vi "Bode plot.vi"(11 "input Bode plot":string) -> (0 "error out":errorcluster, 3 "Bode plot":dbl[][](graph))   [LabVIEW 2020, in "FBN_LATM.lvlib"]
uses:
  FBN_LATM.lvlib
  c2d5c92c-7b70-4316-925e-13b53ebf1ded.vi
  <vilib>/Array/Sort 2D Array - Pop Stack.vi
  <vilib>/Array/Sort 2D Array - Push Stack.vi
  c2d5c92c-7b70-4316-925e-13b53ebf1ded.vi/269d4b3b-47f5-49e3-8884-44851e4dd9d5.vi
  c2d5c92c-7b70-4316-925e-13b53ebf1ded.vi/6d99389c-673d-4efb-bf33-19b32bcf4cf8.vi
  <vilib>/regexp/Match Regular Expression.xnode
panel:
  out "XY Graph":T1(graph)
  out "PosAmpVsCur":dbl[](array[numeric])
  out "PosAmpVsPWM":dbl[](array[numeric])
  out "FreqHz":dbl[](array[numeric])
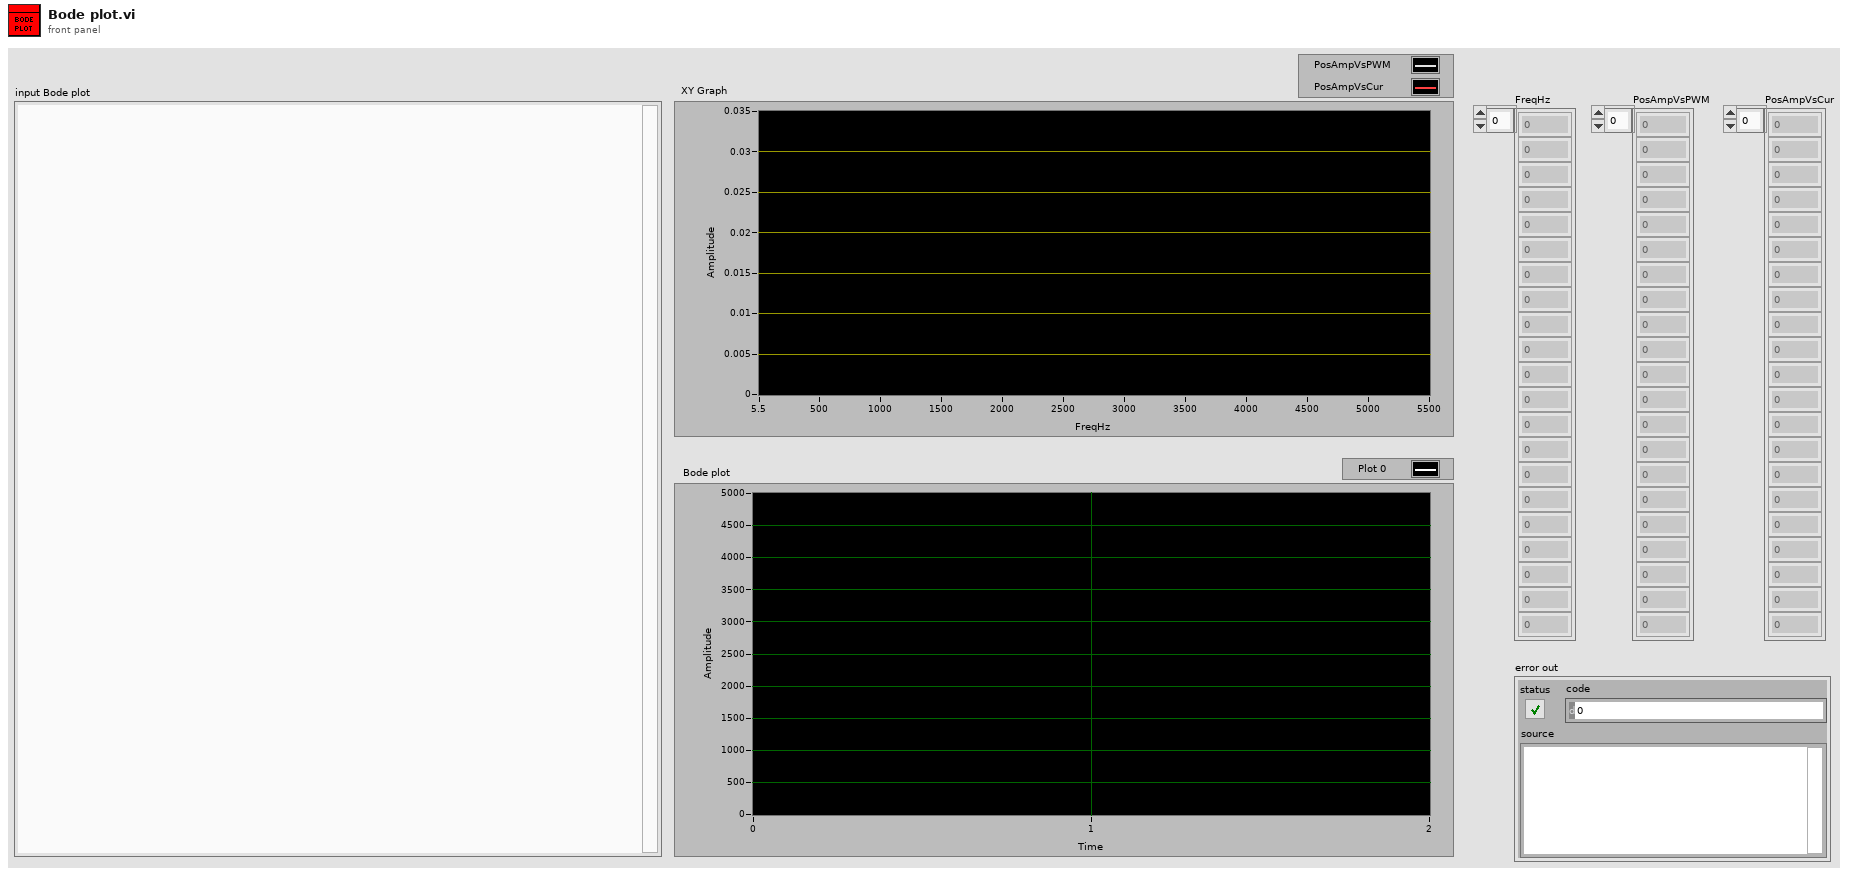
[diagram p1: front panel]
types:
  T1 = cluster{"sorted 2D array":dbl[], "sorted 2D array":dbl[]}[]
  T2 = cluster{"sorted 2D array":dbl[], "sorted 2D array":dbl[]}
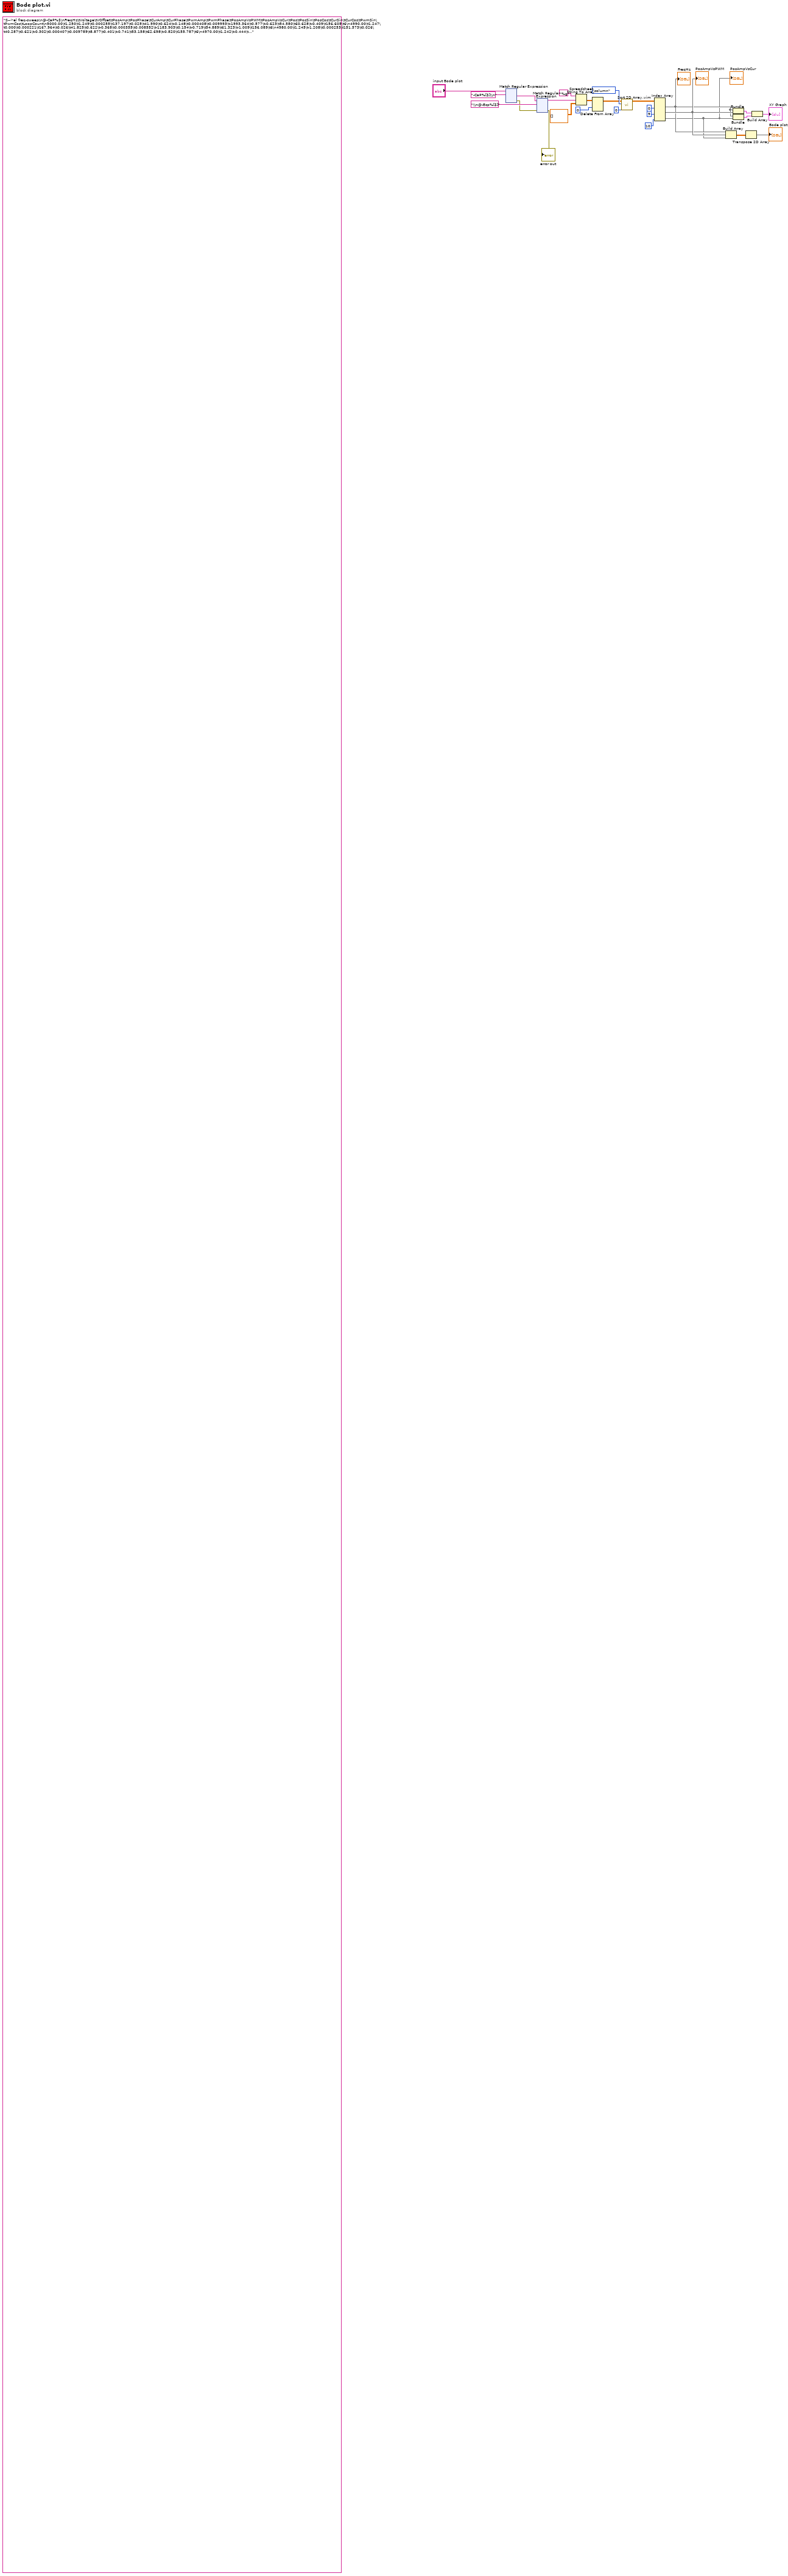
[diagram p0: block diagram]
diagram:
  (unwired) "S-->el freq-sweep\n@-CaP%$\nFreqHz\tVoltage\tVOffset\tPosAmp\tPosPhase\tCurAmp\tCurPhase\tPwmAmp\tPwmPhase\tPosAmpVsPWM\tPosAmpVsCur\tPos\tPosSin\tPosCos\tCurSin\tCurCos\tPwmSin\tPwmCos\tLoopCount\n5000.00\t1.250\t1.249\t0.000255\t137.197\t0.025\t41.990\t0.624\t-0.148\t0.000408\t0.009993\t-1993.364\t0.577\t-0.623\t54.580\t60.628\t-0.409\t156.605\t6\n4990.00\t1.247\t0.000\t0.000221\t167.964\t0.026\t41.825\t0.622\t-0.368\t0.000355\t0.008552\t-1183.903\t0.154\t-0.719\t54.889\t61.323\t-1.009\t156.089\t6\n4980.00\t1.245\t-1.208\t0.000253\t151.573\t0.026\t40.287\t0.621\t-0.302\t0.000407\t0.009789\t8.877\t0.401\t-0.741\t53.158\t62.698\t-0.820\t155.787\t6\n4970.00\t1.242\t-0.444\t0.000163\t148.359\t0.025\t42.056\t0.622\t-0.280\t0.000262\t0.006393\t355.367\t0.285\t-0.462\t54.627\t60.538\t-0.755\t155.800\t6\n4960.00\t1.240\t0.593\t0.000166\t155.248\t0.025\t42.473\t0.620\t-0.313\t0.000268\t0.006519\t341.746\t0.232\t-0.503\t55.286\t60.379\t-0.849\t155.524\t6\n4950.00\t1.237\t-0.866\t0.000154\t154.869\t0.026\t41.006\t0.618\t-0.264\t0.000248\t0.005952\t209.748\t0.218\t-0.464\t54.012\t62.121\t-0.713\t155.158\t6\n4940.00\t1.235\t-0.704\t0.000128\t155.479\t0.025\t41.111\t0.617\t-0.428\t0.000208\t0.005032\t31.794\t0.177\t-0.389\t53.478\t61.286\t-1.155\t154.830\t6\n4930.00\t1.232\t-1.089\t0.000129\t161.532\t0.025\t40.919\t0.615\t-0.330\t0.000209\t0.005050\t8.451\t0.136\t-0.407\t53.623\t61.863\t-0.891\t154.383\t6\n4920.00\t1.230\t-0.495\t0.000107\t155.632\t0.025\t41.869\t0.615\t-0.423\t0.000174\t0.004245\t-76.715\t0.147\t-0.325\t54.031\t60.266\t-1.137\t154.363\t6\n4910.00\t1.227\t1.228\t0.000117\t179.780\t0.026\t42.759\t0.613\t-0.297\t0.000191\t0.004534\t-61.266\t0.002\t-0.390\t55.773\t60.312\t-0.798\t153.814\t6\n4900.00\t1.225\t1.222\t0.000110\t169.025\t0.025\t41.786\t0.612\t-0.346\t0.000179\t0.004351\t-4.380\t0.070\t-0.358\t53.772\t60.160\t-0.925\t153.416\t6\n4890.00\t1.222\t0.000\t0.000144\t178.325\t0.026\t41.468\t0.610\t-0.324\t0.000236\t0.005571\t15.940\t0.014\t-0.479\t54.450\t61.610\t-0.860\t152.959\t6\n4880.00\t1.220\t1.126\t0.000127\t-174.326\t0.025\t41.984\t0.609\t-0.297\t0.000209\t0.004997\t20.182\t-0.042\t-0.422\t54.531\t60.584\t-0.787\t152.760\t6\n4870.00\t1.217\t1.038\t0.000151\t-172.441\t0.026\t42.028\t0.608\t-0.231\t0.000247\t0.005764\t16.908\t-0.066\t-0.498\t55.731\t61.821\t-0.608\t152.596\t6\n4860.00\t1.215\t0.900\t0.000139\t-176.287\t0.025\t41.808\t0.607\t-0.313\t0.000229\t0.005454\t41.706\t-0.030\t-0.462\t54.530\t60.955\t-0.826\t152.379\t6\n4850.00\t1.212\t-0.699\t0.000138\t-165.927\t0.025\t42.484\t0.605\t-0.258\t0.000229\t0.005423\t-5.301\t-0.112\t-0.447\t55.232\t60.289\t-0.682\t151.793\t6\n4840.00\t1.210\t-0.626\t0.000141\t-170.744\t0.026\t42.440\t0.605\t-0.324\t0.000232\t0.005388\t1.882\t-0.075\t-0.463\t56.283\t61.539\t-0.861\t151.883\t6\n4830.00\t1.207\t1.147\t0.000127\t-154.589\t0.025\t42.709\t0.603\t-0.385\t0.000211\t0.004990\t-23.980\t-0.182\t-0.383\t55.051\t59.628\t-1.015\t151.262\t6\n4820.00\t1.205\t0.049\t0.000151\t-162.762\t0.026\t43.033\t0.603\t-0.275\t0.000251\t0.005867\t31.689\t-0.150\t-0.482\t56.139\t60.142\t-0.720\t151.194\t6\n4810.00\t1.202\t-1.186\t0.000142\t-162.048\t0.025\t42.352\t0.601\t-0.412\t0.000236\t0.005624\t21.486\t-0.145\t-0.449\t54.368\t59.627\t-1.089\t150.646\t6\n4800.00\t1.200\t0.196\t0.000150\t-160.373\t0.025\t42.671\t0.600\t-0.269\t0.000249\t0.005866\t33.700\t-0.168\t-0.469\t55.084\t59.751\t-0.698\t150.332\t6\n4790.00\t1.197\t1.095\t0.000173\t-160.378\t0.026\t42.188\t0.597\t-0.269\t0.000290\t0.006714\t10.971\t-0.194\t-0.544\t55.137\t60.813\t-0.701\t149.884\t6\n4780.00\t1.195\t0.835\t0.000152\t-166.388\t0.025\t42.572\t0.597\t-0.291\t0.000254\t0.006026\t-16.344\t-0.119\t-0.491\t54.566\t59.388\t-0.767\t149.810\t6\n4770.00\t1.192\t-0.744\t0.000145\t-156.808\t0.025\t42.880\t0.597\t-0.346\t0.000242\t0.005678\t-13.537\t-0.190\t-0.444\t55.737\t60.020\t-0.905\t149.599\t6\n4760.00\t1.190\t-0.695\t0.000167\t-158.434\t0.026\t42.962\t0.595\t-0.286\t0.000281\t0.006482\t8.466\t-0.205\t-0.518\t56.481\t60.655\t-0.745\t149.185\t6\n4750.00\t1.187\t-1.041\t0.000176\t-159.659\t0.026\t43.500\t0.593\t-0.214\t0.000296\t0.006724\t-22.996\t-0.204\t-0.549\t57.545\t60.632\t-0.555\t148.691\t6\n4740.00\t1.185\t1.182\t0.000181\t-163.098\t0.026\t42.984\t0.592\t-0.231\t0.000306\t0.007017\t0.871\t-0.175\t-0.577\t56.165\t60.271\t-0.599\t148.323\t6\n4730.00\t1.183\t-1.161\t0.000143\t-157.346\t0.025\t44.495\t0.592\t-0.214\t0.000241\t0.005605\t30.673\t-0.183\t-0.440\t56.806\t57.809\t-0.556\t148.407\t6\n4720.00\t1.180\t0.115\t0.000160\t-163.207\t0.025\t43.731\t0.590\t-0.258\t0.000272\t0.006294\t2.617\t-0.155\t-0.512\t56.135\t58.670\t-0.671\t148.080\t6\n4710.00\t1.178\t0.000\t0.000164\t-164.745\t0.025\t44.121\t0.590\t-0.143\t0.000277\t0.006497\t-8.059\t-0.143\t-0.526\t56.342\t58.084\t-0.362\t147.814\t6\n4700.00\t1.175\t-1.164\t0.000155\t-156.242\t0.025\t43.720\t0.587\t-0.346\t0.000263\t0.006062\t3.469\t-0.208\t-0.471\t56.345\t58.904\t-0.886\t147.353\t6\n4690.00\t1.173\t0.000\t0.000177\t-164.910\t0.025\t42.056\t0.587\t-0.214\t0.000302\t0.006960\t-3.623\t-0.154\t-0.571\t54.614\t60.519\t-0.544\t147.385\t6\n4680.00\t1.170\t0.853\t0.000131\t-159.088\t0.025\t43.242\t0.585\t-0.417\t0.000223\t0.005127\t-1.643\t-0.156\t-0.407\t55.531\t59.054\t-1.064\t146.772\t6\n4670.00\t1.168\t-0.688\t0.000177\t-155.803\t0.025\t43.325\t0.583\t-0.236\t0.000304\t0.006948\t-3.205\t-0.242\t-0.538\t55.830\t59.196\t-0.599\t146.292\t6\n4660.00\t1.165\t-1.018\t0.000160\t-154.545\t0.025\t42.720\t0.583\t-0.313\t0.000275\t0.006374\t24.831\t-0.230\t-0.483\t54.934\t59.478\t-0.800\t146.112\t6\n4650.00\t1.163\t0.178\t0.000158\t-149.579\t0.026\t42.951\t0.581\t-0.417\t0.000272\t0.006128\t7.446\t-0.267\t-0.454\t56.012\t60.168\t-1.062\t145.766\t6\n4640.00\t1.160\t0.094\t0.000141\t-155.621\t0.025\t44.028\t0.580\t-0.406\t0.000243\t0.005599\t5.202\t-0.194\t-0.428\t55.760\t57.666\t-1.032\t145.551\t6\n4630.00\t1.158\t0.103\t0.000150\t-156.423\t0.025\t43.209\t0.579\t-0.341\t0.000259\t0.005887\t16.681\t-0.200\t-0.458\t55.817\t59.432\t-0.868\t145.294\t6\n4620.00\t1.155\t1.155\t0.000182\t-153.858\t0.026\t42.715\t0.578\t-0.297\t0.000315\t0.007058\t46.128\t-0.268\t-0.545\t55.730\t60.355\t-0.745\t144.788\t6\n4610.00\t1.153\t-0.619\t0.000159\t-155.132\t0.025\t44.764\t0.577\t-0.302\t0.000276\t0.006331\t16.596\t-0.224\t-0.482\t56.336\t56.801\t-0.757\t144.661\t6\n4600.00\t1.150\t-0.613\t0.000185\t-157.214\t0.025\t44.621\t0.575\t-0.319\t0.000323\t0.007276\t-14.436\t-0.239\t-0.570\t57.219\t57.971\t-0.808\t144.317\t6\n4590.00\t1.148\t0.831\t0.000185\t-148.211\t0.025\t45.093\t0.574\t-0.253\t0.000323\t0.007352\t22.962\t-0.325\t-0.524\t57.075\t56.877\t-0.636\t143.873\t6\n4580.00\t1.145\t0.899\t0.000161\t-151.941\t0.025\t44.247\t0.573\t-0.352\t0.000281\t0.006315\t26.916\t-0.253\t-0.474\t56.586\t58.077\t-0.883\t143.620\t6\n4570.00\t1.143\t0.000\t0.000167\t-156.423\t0.025\t44.094\t0.571\t-0.280\t0.000292\t0.006714\t12.777\t-0.222\t-0.510\t55.435\t57.206\t-0.698\t143.261\t6\n4560.00\t1.140\t1.140\t0.000178\t-148.870\t0.025\t45.143\t0.570\t-0.291\t0.000312\t0.007051\t-20.910\t-0.306\t-0.506\t57.204\t56.911\t-0.722\t143.006\t6\n4550.00\t1.138\t0.206\t0.000173\t-156.907\t0.025\t43.912\t0.569\t-0.368\t0.000304\t0.006781\t-28.046\t-0.226\t-0.530\t56.208\t58.365\t-0.921\t142.743\t6\n4540.00\t1.135\t-1.106\t0.000174\t-152.292\t0.025\t44.253\t0.568\t-0.357\t0.000306\t0.006992\t4.846\t-0.270\t-0.513\t55.734\t57.196\t-0.887\t142.371\t6\n4530.00\t1.133\t-0.389\t0.000175\t-148.788\t0.025\t45.192\t0.567\t-0.313\t0.000308\t0.006846\t23.396\t-0.302\t-0.498\t57.768\t57.377\t-0.769\t142.138\t6\n4520.00\t1.130\t-1.108\t0.000164\t-151.523\t0.025\t45.088\t0.565\t-0.412\t0.000291\t0.006521\t27.756\t-0.261\t-0.481\t57.160\t56.972\t-1.016\t141.756\t6\n4510.00\t1.128\t0.836\t0.000181\t-150.249\t0.025\t44.594\t0.564\t-0.319\t0.000321\t0.007192\t8.173\t-0.300\t-0.524\t56.858\t57.664\t-0.791\t141.476\t6\n4500.00\t1.125\t0.808\t0.000165\t-150.408\t0.025\t46.082\t0.563\t-0.214\t0.000293\t0.006564\t6.295\t-0.272\t-0.479\t58.289\t56.146\t-0.522\t141.321\t6\n4490.00\t1.122\t0.925\t0.000214\t-149.227\t0.025\t45.005\t0.560\t-0.214\t0.000382\t0.008509\t-15.610\t-0.366\t-0.613\t57.208\t57.214\t-0.524\t140.490\t6\n4480.00\t1.120\t-1.072\t0.000164\t-151.996\t0.025\t45.082\t0.560\t-0.291\t0.000293\t0.006533\t-28.654\t-0.258\t-0.484\t57.342\t57.163\t-0.719\t140.568\t6\n4470.00\t1.117\t-0.601\t0.000186\t-153.166\t0.025\t45.994\t0.559\t-0.297\t0.000333\t0.007498\t-31.188\t-0.281\t-0.554\t56.969\t55.035\t-0.727\t140.307\t6\n4460.00\t1.115\t1.114\t0.000163\t-153.715\t0.025\t45.522\t0.560\t-0.363\t0.000291\t0.006459\t3.896\t-0.240\t-0.486\t57.659\t56.629\t-0.882\t140.291\t6\n4450.00\t1.112\t0.000\t0.000163\t-148.057\t0.025\t45.582\t0.558\t-0.434\t0.000293\t0.006487\t36.432\t-0.288\t-0.462\t57.528\t56.384\t-1.064\t139.899\t6\n4440.00\t1.110\t-1.088\t0.000177\t-155.006\t0.025\t45.753\t0.555\t-0.330\t0.000320\t0.007047\t12.589\t-0.250\t-0.536\t57.923\t56.436\t-0.796\t139.268\t6\n4430.00\t1.107\t-1.041\t0.000163\t-154.363\t0.025\t44.604\t0.554\t-0.483\t0.000294\t0.006470\t10.345\t-0.235\t-0.490\t56.292\t57.068\t-1.168\t138.921\t6\n4420.00\t1.105\t0.833\t0.000164\t-157.972\t0.025\t45.379\t0.553\t-0.330\t0.000296\t0.006511\t19.977\t-0.205\t-0.506\t57.381\t56.631\t-0.793\t138.906\t6\n4410.00\t1.102\t0.000\t0.000167\t-154.869\t0.025\t44.890\t0.552\t-0.275\t0.000303\t0.006647\t14.153\t-0.237\t-0.505\t57.051\t57.276\t-0.668\t138.555\t6\n4400.00\t1.100\t-0.377\t0.000142\t-157.791\t0.025\t46.384\t0.551\t-0.385\t0.000258\t0.005657\t-16.028\t-0.179\t-0.440\t58.265\t55.519\t-0.923\t138.310\t6\n4390.00\t1.097\t-1.048\t0.000168\t-154.951\t0.025\t45.753\t0.549\t-0.308\t0.000306\t0.006682\t-37.026\t-0.237\t-0.508\t58.000\t56.513\t-0.734\t137.758\t6\n4380.00\t1.095\t0.000\t0.000152\t-153.583\t0.025\t45.961\t0.548\t-0.385\t0.000278\t0.006054\t-23.497\t-0.226\t-0.455\t57.690\t55.796\t-0.926\t137.567\t6\n4370.00\t1.092\t0.000\t0.000147\t-156.528\t0.025\t46.604\t0.547\t-0.412\t0.000268\t0.005820\t-9.884\t-0.195\t-0.448\t58.351\t55.167\t-0.989\t137.263\t6\n4360.00\t1.090\t0.071\t0.000155\t-150.650\t0.025\t45.599\t0.547\t-0.417\t0.000284\t0.006165\t18.959\t-0.254\t-0.451\t57.755\t56.569\t-0.998\t137.186\t6\n4350.00\t1.087\t-0.637\t0.000165\t-150.040\t0.025\t46.208\t0.544\t-0.390\t0.000303\t0.006644\t19.041\t-0.275\t-0.477\t57.424\t55.067\t-0.925\t136.610\t6\n4340.00\t1.085\t-0.560\t0.000171\t-154.341\t0.025\t46.703\t0.544\t-0.341\t0.000314\t0.006782\t16.913\t-0.246\t-0.513\t58.281\t54.913\t-0.807\t136.437\t6\n4330.00\t1.082\t1.064\t0.000156\t-153.754\t0.025\t46.851\t0.541\t-0.363\t0.000288\t0.006276\t33.703\t-0.230\t-0.466\t57.833\t54.203\t-0.861\t135.875\t6\n4320.00\t1.080\t-0.585\t0.000163\t-153.979\t0.025\t46.137\t0.542\t-0.352\t0.000300\t0.006546\t12.338\t-0.238\t-0.487\t57.525\t55.298\t-0.838\t135.724\t6\n4310.00\t1.077\t0.860\t0.000179\t-152.139\t0.025\t47.137\t0.540\t-0.346\t0.000332\t0.007124\t-4.306\t-0.280\t-0.528\t59.237\t54.972\t-0.814\t135.397\t6\n4300.00\t1.075\t-1.026\t0.000183\t-154.177\t0.025\t47.324\t0.539\t-0.269\t0.000339\t0.007353\t-1.340\t-0.266\t-0.548\t58.630\t54.066\t-0.636\t135.062\t6\n4290.00\t1.072\t-0.633\t0.000177\t-157.665\t0.025\t47.752\t0.537\t-0.286\t0.000329\t0.007021\t-7.997\t-0.224\t-0.545\t59.389\t53.958\t-0.674\t134.707\t6\n4280.00\t1.070\t1.068\t0.000183\t-156.885\t0.025\t47.648\t0.536\t-0.341\t0.000341\t0.007179\t-12.853\t-0.239\t-0.561\t59.862\t54.584\t-0.795\t134.490\t6\n4270.00\t1.067\t1.052\t0.000181\t-158.329\t0.025\t47.873\t0.535\t-0.242\t0.000338\t0.007378\t-2.887\t-0.223\t-0.561\t58.349\t52.786\t-0.563\t134.174\t6\n4260.00\t1.065\t-0.975\t0.000191\t-167.135\t0.025\t47.994\t0.534\t-0.137\t0.000358\t0.007791\t2.205\t-0.142\t-0.621\t58.549\t52.749\t-0.324\t134.071\t6\n4250.00\t1.062\t0.763\t0.000177\t-164.685\t0.025\t47.791\t0.533\t-0.209\t0.000333\t0.007036\t18.626\t-0.156\t-0.569\t59.454\t53.944\t-0.491\t133.578\t6\n4240.00\t1.060\t0.000\t0.000193\t-164.317\t0.025\t48.010\t0.531\t-0.253\t0.000363\t0.007573\t3.350\t-0.174\t-0.620\t60.480\t54.447\t-0.587\t133.155\t6\n4230.00\t1.058\t0.908\t0.000160\t-165.482\t0.025\t48.263\t0.530\t-0.154\t0.000301\t0.006425\t-6.285\t-0.134\t-0.515\t59.474\t53.068\t-0.355\t133.034\t6\n4220.00\t1.055\t-0.447\t0.000163\t176.094\t0.025\t47.005\t0.531\t-0.214\t0.000307\t0.006555\t-12.677\t0.037\t-0.542\t58.274\t54.325\t-0.497\t133.300\t6\n4210.00\t1.053\t0.071\t0.000153\t-176.561\t0.025\t46.934\t0.529\t-0.297\t0.000289\t0.005989\t-9.868\t-0.031\t-0.508\t59.400\t55.515\t-0.692\t132.757\t6\n4200.00\t1.050\t1.048\t0.000154\t175.649\t0.025\t47.994\t0.529\t-0.082\t0.000291\t0.006202\t0.065\t0.039\t-0.512\t59.155\t53.294\t-0.193\t132.717\t6\n4190.00\t1.048\t0.337\t0.000136\t169.146\t0.025\t48.505\t0.529\t-0.192\t0.000258\t0.005480\t25.157\t0.086\t-0.446\t59.712\t52.827\t-0.446\t132.497\t6\n4180.00\t1.045\t0.000\t0.000110\t156.028\t0.025\t47.450\t0.529\t-0.406\t0.000207\t0.004411\t23.464\t0.149\t-0.334\t58.879\t54.061\t-0.941\t132.635\t6\n4170.00\t1.043\t-0.971\t0.000083\t152.650\t0.025\t47.818\t0.528\t-0.516\t0.000156\t0.003280\t11.400\t0.127\t-0.245\t59.347\t53.790\t-1.197\t132.399\t6\n4160.00\t1.040\t0.525\t0.000054\t154.358\t0.025\t47.565\t0.527\t-0.709\t0.000103\t0.002134\t-15.810\t0.079\t-0.164\t59.980\t54.853\t-1.633\t132.092\t6\n4150.00\t1.038\t0.822\t0.000029\t139.823\t0.025\t47.395\t0.526\t-0.807\t0.000055\t0.001140\t-13.850\t0.062\t-0.074\t59.880\t55.081\t-1.857\t131.983\t6\n4140.00\t1.035\t0.000\t0.000028\t-61.935\t0.025\t47.406\t0.522\t-1.143\t0.000054\t0.001128\t4.198\t-0.083\t0.044\t58.388\t53.687\t-2.616\t130.956\t6\n4130.00\t1.033\t0.000\t0.000038\t-55.497\t0.025\t46.637\t0.522\t-1.121\t0.000074\t0.001506\t-1.633\t-0.106\t0.072\t59.033\t55.744\t-2.569\t131.014\t6\n4120.00\t1.030\t-0.977\t0.000089\t-54.904\t0.025\t47.302\t0.519\t-1.230\t0.000172\t0.003599\t7.216\t-0.244\t0.172\t58.374\t53.870\t-2.799\t130.155\t6\n4110.00\t1.028\t-0.571\t0.000125\t-64.270\t0.025\t46.659\t0.516\t-1.373\t0.000243\t0.005043\t30.846\t-0.377\t0.181\t57.990\t54.717\t-3.110\t129.443\t6\n4100.00\t1.025\t0.206\t0.000177\t-72.647\t0.024\t46.818\t0.511\t-1.472\t0.000346\t0.007308\t23.431\t-0.563\t0.176\t56.761\t53.252\t-3.297\t128.255\t6\n4090.00\t1.023\t1.014\t0.000209\t-90.000\t0.025\t47.230\t0.508\t-1.313\t0.000410\t0.008386\t8.200\t-0.695\t0.000\t58.240\t53.881\t-2.925\t127.445\t6\n4080.00\t1.020\t0.462\t0.000269\t-101.580\t0.025\t46.362\t0.504\t-1.066\t0.000533\t0.010953\t-9.971\t-0.878\t-0.180\t56.859\t54.220\t-2.361\t126.591\t6\n4070.00\t1.018\t0.000\t0.000313\t-115.203\t0.024\t47.670\t0.502\t-0.593\t0.000623\t0.012904\t-30.148\t-0.943\t-0.444\t57.179\t52.100\t-1.302\t125.957\t6\n4060.00\t1.015\t0.814\t0.000293\t-128.057\t0.024\t48.977\t0.503\t-0.445\t0.000583\t0.012267\t-31.429\t-0.770\t-0.603\t57.390\t49.920\t-0.982\t126.131\t6\n4050.00\t1.013\t0.000\t0.000302\t-137.922\t0.025\t48.697\t0.501\t-0.247\t0.000603\t0.012317\t-5.351\t-0.675\t-0.748\t58.643\t51.521\t-0.536\t125.787\t6\n4040.00\t1.010\t-0.442\t0.000291\t-153.776\t0.025\t49.850\t0.504\t0.038\t0.000578\t0.011866\t16.688\t-0.429\t-0.871\t59.651\t50.332\t0.080\t126.375\t6\n4030.00\t1.008\t0.027\t0.000267\t-162.488\t0.025\t48.796\t0.505\t0.060\t0.000529\t0.010886\t30.221\t-0.268\t-0.850\t58.884\t51.545\t0.130\t126.608\t6\n4020.00\t1.005\t1.001\t0.000229\t-170.815\t0.025\t49.570\t0.506\t-0.104\t0.000453\t0.009216\t8.998\t-0.122\t-0.754\t60.337\t51.420\t-0.227\t126.879\t6\n4010.00\t1.003\t0.221\t0.000147\t-175.391\t0.025\t49.136\t0.506\t-0.472\t0.000291\t0.005858\t-2.574\t-0.040\t-0.490\t61.009\t52.784\t-1.040\t126.861\t6\n4000.00\t1.000\t0.264\t0.000143\t-159.208\t0.025\t49.883\t0.503\t-0.467\t0.000285\t0.005763\t-54.212\t-0.170\t-0.446\t61.031\t51.441\t-1.032\t126.112\t6\n3990.00\t0.998\t0.000\t0.000152\t-159.373\t0.025\t48.329\t0.501\t-0.571\t0.000302\t0.006176\t39.815\t-0.178\t-0.473\t58.889\t52.423\t-1.252\t125.767\t6\n3980.00\t0.995\t0.671\t0.000151\t-165.547\t0.025\t49.103\t0.501\t-0.423\t0.000303\t0.006171\t7.793\t-0.126\t-0.489\t59.676\t51.687\t-0.922\t125.646\t6\n3970.00\t0.993\t0.000\t0.000155\t-162.059\t0.025\t49.477\t0.500\t-0.478\t0.000311\t0.006247\t-13.182\t-0.160\t-0.492\t60.675\t51.871\t-1.040\t125.344\t6\n3960.00\t0.990\t-0.324\t0.000134\t-162.493\t0.025\t49.164\t0.497\t-0.604\t0.000269\t0.005377\t-13.535\t-0.134\t-0.425\t60.097\t51.945\t-1.315\t124.843\t6\n3950.00\t0.988\t0.000\t0.000121\t-156.671\t0.025\t49.449\t0.497\t-0.637\t0.000244\t0.004875\t19.172\t-0.160\t-0.371\t60.052\t51.390\t-1.388\t124.631\t6\n3940.00\t0.985\t0.000\t0.000114\t-167.943\t0.025\t49.724\t0.497\t-0.698\t0.000230\t0.004590\t16.340\t-0.080\t-0.372\t60.546\t51.320\t-1.514\t124.576\t6\n3930.00\t0.983\t0.213\t0.000136\t-161.494\t0.025\t49.449\t0.495\t-0.577\t0.000274\t0.005385\t-3.933\t-0.143\t-0.429\t61.120\t52.309\t-1.252\t124.055\t6\n3920.00\t0.980\t0.971\t0.000125\t-158.610\t0.025\t50.246\t0.493\t-0.725\t0.000253\t0.005093\t-40.909\t-0.152\t-0.388\t60.201\t50.088\t-1.567\t123.686\t6\n3910.00\t0.978\t0.000\t0.000100\t-153.160\t0.025\t49.362\t0.492\t-0.928\t0.000203\t0.004023\t-13.336\t-0.150\t-0.298\t60.033\t51.536\t-1.997\t123.346\t6\n3900.00\t0.975\t-0.904\t0.000106\t-158.044\t0.025\t49.241\t0.490\t-0.901\t0.000217\t0.004329\t32.541\t-0.133\t-0.329\t59.795\t51.542\t-1.932\t123.007\t6\n3890.00\t0.973\t-0.468\t0.000104\t-152.589\t0.024\t50.015\t0.489\t-0.862\t0.000212\t0.004275\t23.589\t-0.159\t-0.306\t59.468\t49.888\t-1.844\t122.692\t6\n3880.00\t0.970\t0.000\t0.000112\t-158.038\t0.025\t49.905\t0.488\t-0.884\t0.000230\t0.004573\t12.163\t-0.140\t-0.347\t59.871\t50.425\t-1.892\t122.564\t6\n3870.00\t0.967\t-0.226\t0.000093\t-145.745\t0.025\t49.504\t0.486\t-0.950\t0.000192\t0.003800\t0.454\t-0.175\t-0.257\t59.794\t51.073\t-2.023\t121.864\t6\n3860.00\t0.965\t-0.436\t0.000102\t-154.792\t0.025\t50.312\t0.485\t-0.895\t0.000211\t0.004174\t-1.191\t-0.145\t-0.309\t60.726\t50.404\t-1.906\t121.680\t6\n3850.00\t0.962\t0.461\t0.000114\t-154.660\t0.025\t49.757\t0.484\t-0.873\t0.000235\t0.004638\t-1.584\t-0.163\t-0.343\t59.813\t50.635\t-1.848\t121.318\t6\n3840.00\t0.960\t-0.638\t0.000107\t-143.811\t0.025\t50.257\t0.481\t-0.956\t0.000222\t0.004291\t1.456\t-0.210\t-0.287\t61.062\t50.784\t-2.017\t120.790\t6\n3830.00\t0.957\t0.949\t0.000100\t-158.143\t0.025\t50.570\t0.482\t-0.945\t0.000207\t0.004018\t0.609\t-0.124\t-0.309\t61.039\t50.190\t-1.998\t120.826\t6\n3820.00\t0.955\t-0.030\t0.000094\t-146.777\t0.025\t50.944\t0.479\t-1.022\t0.000195\t0.003813\t2.689\t-0.171\t-0.261\t60.948\t49.440\t-2.143\t120.213\t6\n3810.00\t0.952\t0.000\t0.000091\t-148.881\t0.025\t50.372\t0.478\t-1.038\t0.000191\t0.003712\t-13.233\t-0.157\t-0.260\t60.524\t50.130\t-2.173\t119.907\t6\n3800.00\t0.950\t0.764\t0.000083\t-147.008\t0.025\t49.406\t0.477\t-1.077\t0.000174\t0.003388\t18.961\t-0.151\t-0.233\t59.539\t51.030\t-2.254\t119.676\t6\n3790.00\t0.947\t0.000\t0.000091\t-147.101\t0.025\t50.350\t0.476\t-1.055\t0.000191\t0.003712\t16.231\t-0.165\t-0.255\t60.586\t50.216\t-2.197\t119.397\t6\n3780.00\t0.945\t0.000\t0.000082\t-140.081\t0.025\t48.774\t0.474\t-1.198\t0.000172\t0.003281\t11.820\t-0.175\t-0.208\t59.719\t52.321\t-2.486\t118.968\t6\n3770.00\t0.942\t-0.647\t0.000074\t-145.020\t0.025\t50.295\t0.473\t-1.137\t0.000156\t0.003006\t-8.819\t-0.141\t-0.202\t60.630\t50.351\t-2.357\t118.784\t6\n3760.00\t0.940\t-0.638\t0.000074\t-135.159\t0.025\t50.850\t0.472\t-1.192\t0.000158\t0.003033\t-19.094\t-0.175\t-0.176\t60.560\t49.289\t-2.463\t118.281\t6\n3750.00\t0.937\t0.000\t0.000032\t-148.217\t0.025\t51.048\t0.470\t-1.252\t0.000069\t0.001323\t-5.418\t-0.057\t-0.092\t60.981\t49.286\t-2.575\t117.902\t6\n3740.00\t0.935\t0.462\t0.000063\t-141.235\t0.024\t50.098\t0.469\t-1.296\t0.000133\t0.002580\t-5.761\t-0.131\t-0.163\t59.739\t49.969\t-2.663\t117.640\t6\n3730.00\t0.933\t-0.747\t0.000059\t-151.935\t0.025\t50.603\t0.469\t-1.241\t0.000125\t0.002389\t-11.749\t-0.092\t-0.172\t60.509\t49.698\t-2.548\t117.545\t6\n3720.00\t0.930\t0.000\t0.000047\t-152.622\t0.025\t50.817\t0.468\t-1.368\t0.000100\t0.001889\t11.241\t-0.072\t-0.139\t61.266\t49.925\t-2.801\t117.394\t6\n3710.00\t0.928\t-0.434\t0.000057\t-123.558\t0.025\t49.686\t0.465\t-1.357\t0.000123\t0.002332\t11.339\t-0.159\t-0.106\t59.862\t50.801\t-2.763\t116.521\t6\n3700.00\t0.925\t-0.389\t0.000048\t-131.732\t0.024\t50.966\t0.464\t-1.412\t0.000105\t0.001999\t27.426\t-0.120\t-0.108\t60.144\t48.749\t-2.862\t116.234\t6\n3690.00\t0.923\t0.000\t0.000045\t-141.130\t0.025\t51.092\t0.462\t-1.417\t0.000097\t0.001798\t-2.266\t-0.093\t-0.116\t62.059\t50.086\t-2.867\t115.894\t6\n3680.00\t0.920\t-0.429\t0.000018\t-170.387\t0.024\t50.048\t0.461\t-1.577\t0.000039\t0.000751\t-30.753\t-0.010\t-0.059\t58.264\t48.821\t-3.187\t115.677\t6\n3670.00\t0.918\t-0.856\t0.000027\t-149.546\t0.025\t50.674\t0.459\t-1.549\t0.000058\t0.001085\t-11.408\t-0.045\t-0.077\t60.748\t49.761\t-3.116\t115.272\t6\n3660.00\t0.915\t0.000\t0.000009\t-113.198\t0.024\t50.026\t0.458\t-1.681\t0.000020\t0.000382\t31.722\t-0.028\t-0.012\t58.975\t49.450\t-3.377\t114.888\t6\n3650.00\t0.913\t0.000\t0.000016\t-43.083\t0.025\t50.328\t0.457\t-1.626\t0.000035\t0.000644\t18.317\t-0.036\t0.039\t60.211\t49.943\t-3.252\t114.418\t6\n3640.00\t0.910\t0.000\t0.000030\t-27.208\t0.024\t50.482\t0.455\t-1.747\t0.000066\t0.001232\t5.719\t-0.045\t0.088\t59.907\t49.421\t-3.479\t114.003\t6\n3630.00\t0.908\t0.795\t0.000033\t-26.340\t0.024\t50.175\t0.453\t-1.747\t0.000074\t0.001381\t1.122\t-0.050\t0.100\t59.862\t49.931\t-3.465\t113.555\t6\n3620.00\t0.905\t0.000\t0.000064\t-5.400\t0.024\t50.861\t0.452\t-1.978\t0.000141\t0.002700\t16.423\t-0.020\t0.212\t58.771\t47.817\t-3.913\t113.200\t6\n3610.00\t0.902\t0.606\t0.000079\t0.544\t0.024\t50.312\t0.450\t-2.071\t0.000176\t0.003318\t0.571\t0.003\t0.265\t59.102\t49.057\t-4.076\t112.763\t6\n3600.00\t0.900\t0.783\t0.000079\t-7.883\t0.024\t51.279\t0.448\t-1.956\t0.000176\t0.003292\t-3.072\t-0.036\t0.260\t60.069\t48.164\t-3.837\t112.331\t6\n3590.00\t0.897\t0.532\t0.000094\t12.288\t0.025\t50.598\t0.448\t-2.115\t0.000211\t0.003846\t-16.253\t0.067\t0.308\t60.450\t49.657\t-4.152\t112.355\t6\n3580.00\t0.895\t0.000\t0.000139\t-4.142\t0.024\t49.850\t0.444\t-2.450\t0.000313\t0.005741\t-2.114\t-0.034\t0.462\t59.567\t50.264\t-4.768\t111.358\t6\n3570.00\t0.892\t0.000\t0.000175\t-5.795\t0.024\t50.790\t0.442\t-2.510\t0.000396\t0.007230\t-11.565\t-0.059\t0.581\t60.019\t48.959\t-4.858\t110.784\t6\n3560.00\t0.890\t0.471\t0.000227\t-3.340\t0.024\t49.883\t0.439\t-2.659\t0.000516\t0.009600\t-17.143\t-0.044\t0.754\t57.706\t48.639\t-5.112\t110.041\t6\n3550.00\t0.887\t0.561\t0.000292\t-12.574\t0.024\t51.246\t0.435\t-2.653\t0.000671\t0.012372\t-13.186\t-0.212\t0.950\t59.089\t47.437\t-5.053\t109.087\t6\n3540.00\t0.885\t0.746\t0.000310\t-14.650\t0.023\t50.191\t0.431\t-2.834\t0.000718\t0.013295\t24.523\t-0.261\t0.999\t57.317\t47.778\t-5.350\t107.969\t6\n3530.00\t0.882\t-0.571\t0.000360\t-18.391\t0.023\t49.065\t0.427\t-2.856\t0.000843\t0.015449\t35.429\t-0.379\t1.138\t56.536\t49.033\t-5.336\t106.989\t6\n3520.00\t0.880\t-0.311\t0.000469\t-25.137\t0.023\t49.702\t0.421\t-2.763\t0.001113\t0.020688\t11.536\t-0.664\t1.415\t55.230\t46.850\t-5.092\t105.516\t6\n3510.00\t0.877\t0.000\t0.000523\t-35.189\t0.023\t50.411\t0.416\t-2.499\t0.001256\t0.023086\t-1.065\t-1.005\t1.425\t56.055\t46.365\t-4.553\t104.356\t6\n3500.00\t0.875\t0.000\t0.000562\t-44.566\t0.022\t50.136\t0.413\t-1.912\t0.001363\t0.025168\t-35.347\t-1.315\t1.335\t55.236\t46.135\t-3.454\t103.441\t6\n3490.00\t0.873\t-0.282\t0.000599\t-56.398\t0.023\t50.718\t0.409\t-1.181\t0.001464\t0.026453\t-22.756\t-1.664\t1.106\t55.904\t45.721\t-2.116\t102.641\t6\n3480.00\t0.870\t0.021\t0.000653\t-65.748\t0.022\t53.586\t0.409\t-0.472\t0.001598\t0.029656\t-13.737\t-1.985\t0.894\t56.407\t41.613\t-0.849\t102.521\t6\n3470.00\t0.868\t0.864\t0.000633\t-76.877\t0.023\t53.157\t0.410\t0.126\t0.001543\t0.027924\t-37.774\t-2.054\t0.479\t57.725\t43.237\t0.229\t102.815\t6\n3460.00\t0.865\t0.188\t0.000607\t-83.990\t0.022\t54.613\t0.412\t0.571\t0.001474\t0.027169\t-22.587\t-2.013\t0.212\t58.050\t41.249\t1.034\t103.322\t6\n3450.00\t0.863\t0.777\t0.000573\t-89.698\t0.023\t54.223\t0.413\t0.648\t0.001386\t0.025268\t1.833\t-1.908\t0.010\t58.766\t42.363\t1.175\t103.531\t6\n3440.00\t0.860\t0.475\t0.000544\t-96.790\t0.022\t54.739\t0.415\t0.764\t0.001310\t0.024365\t23.878\t-1.802\t-0.214\t58.441\t41.331\t1.388\t104.257\t6\n3430.00\t0.858\t0.586\t0.000527\t-101.497\t0.023\t54.388\t0.416\t0.890\t0.001266\t0.022927\t23.715\t-1.720\t-0.350\t59.748\t42.809\t1.618\t104.431\t6\n3420.00\t0.855\t0.000\t0.000505\t-106.705\t0.023\t54.080\t0.417\t0.873\t0.001209\t0.021964\t24.901\t-1.611\t-0.483\t59.724\t43.276\t1.599\t104.649\t6\n3410.00\t0.853\t0.000\t0.000478\t-109.715\t0.023\t55.750\t0.418\t0.840\t0.001143\t0.020801\t-12.084\t-1.500\t-0.537\t60.510\t41.201\t1.532\t104.802\t6\n3400.00\t0.850\t-0.290\t0.000458\t-115.181\t0.023\t54.591\t0.418\t0.802\t0.001095\t0.019673\t-9.374\t-1.382\t-0.650\t60.819\t43.245\t1.471\t104.968\t6\n3390.00\t0.848\t-0.728\t0.000433\t-112.115\t0.023\t55.920\t0.417\t0.654\t0.001037\t0.018571\t11.990\t-1.335\t-0.543\t62.035\t41.975\t1.197\t104.625\t6\n3380.00\t0.845\t0.535\t0.000400\t-117.795\t0.023\t55.734\t0.418\t0.555\t0.000958\t0.017192\t8.798\t-1.181\t-0.623\t61.850\t42.137\t1.012\t104.838\t6\n3370.00\t0.842\t0.803\t0.000371\t-114.807\t0.024\t54.998\t0.416\t0.209\t0.000893\t0.015732\t-2.975\t-1.123\t-0.519\t62.243\t43.589\t0.375\t104.304\t6\n3360.00\t0.840\t0.000\t0.000345\t-115.378\t0.024\t54.014\t0.416\t0.044\t0.000830\t0.014631\t7.435\t-1.040\t-0.493\t60.819\t44.176\t0.077\t104.350\t6\n3350.00\t0.837\t0.298\t0.000388\t-120.383\t0.024\t55.657\t0.415\t0.500\t0.000935\t0.016444\t5.559\t-1.116\t-0.654\t62.080\t42.411\t0.907\t104.126\t6\n3340.00\t0.835\t0.000\t0.000369\t-115.917\t0.023\t54.245\t0.412\t0.110\t0.000895\t0.015841\t-24.978\t-1.106\t-0.537\t60.349\t43.465\t0.201\t103.312\t6\n3330.00\t0.832\t-0.095\t0.000369\t-119.938\t0.023\t54.619\t0.411\t0.297\t0.000897\t0.015847\t-29.241\t-1.066\t-0.614\t60.957\t43.301\t0.536\t103.412\t6\n3320.00\t0.830\t0.416\t0.000358\t-121.668\t0.023\t56.354\t0.412\t0.253\t0.000870\t0.015385\t-24.126\t-1.016\t-0.627\t62.158\t41.378\t0.451\t103.195\t6\n3310.00\t0.827\t-0.299\t0.000353\t-124.464\t0.024\t55.459\t0.412\t0.203\t0.000858\t0.014960\t9.598\t-0.970\t-0.666\t61.861\t42.568\t0.368\t103.225\t6\n3300.00\t0.825\t0.000\t0.000340\t-122.794\t0.023\t54.937\t0.409\t0.154\t0.000831\t0.014589\t18.020\t-0.952\t-0.613\t61.371\t43.077\t0.278\t102.620\t6\n3290.00\t0.822\t0.000\t0.000329\t-123.398\t0.023\t56.250\t0.409\t0.011\t0.000805\t0.014120\t23.819\t-0.915\t-0.604\t62.181\t41.559\t0.019\t102.543\t6\n3280.00\t0.820\t0.041\t0.000319\t-127.244\t0.024\t55.783\t0.408\t0.121\t0.000782\t0.013524\t30.510\t-0.847\t-0.644\t62.136\t42.255\t0.218\t102.451\t6\n3270.00\t0.817\t-0.740\t0.000313\t-126.359\t0.023\t55.772\t0.406\t0.038\t0.000770\t0.013437\t12.427\t-0.840\t-0.618\t61.805\t42.045\t0.071\t102.011\t6\n3260.00\t0.815\t0.275\t0.000297\t-125.942\t0.024\t56.025\t0.406\t-0.066\t0.000731\t0.012568\t13.075\t-0.800\t-0.580\t62.660\t42.235\t-0.120\t101.693\t6\n3250.00\t0.812\t0.564\t0.000295\t-123.799\t0.023\t55.794\t0.403\t-0.143\t0.000731\t0.012665\t-5.464\t-0.817\t-0.547\t61.972\t42.124\t-0.254\t101.234\t6\n3240.00\t0.810\t0.646\t0.000294\t-127.711\t0.023\t54.415\t0.404\t-0.115\t0.000730\t0.012645\t2.204\t-0.776\t-0.600\t60.972\t43.641\t-0.199\t101.241\t6\n3230.00\t0.808\t-0.779\t0.000284\t-125.310\t0.023\t54.278\t0.401\t-0.181\t0.000707\t0.012527\t-7.227\t-0.772\t-0.547\t59.107\t42.524\t-0.322\t100.692\t6\n3220.00\t0.805\t0.000\t0.000281\t-122.558\t0.023\t56.503\t0.400\t-0.176\t0.000701\t0.012051\t-5.995\t-0.788\t-0.503\t62.036\t41.074\t-0.302\t100.368\t6\n3210.00\t0.803\t0.039\t0.000272\t-125.277\t0.024\t55.865\t0.399\t-0.192\t0.000682\t0.011530\t14.107\t-0.741\t-0.524\t62.685\t42.495\t-0.339\t100.082\t6\n3200.00\t0.800\t-0.206\t0.000264\t-124.140\t0.024\t55.410\t0.397\t-0.286\t0.000663\t0.011164\t17.985\t-0.727\t-0.493\t61.765\t42.583\t-0.491\t99.676\t6\n3190.00\t0.798\t-0.576\t0.000249\t-120.366\t0.023\t56.096\t0.396\t-0.308\t0.000630\t0.011011\t10.194\t-0.717\t-0.420\t60.533\t40.689\t-0.534\t99.260\t6\n3180.00\t0.795\t-0.768\t0.000251\t-115.933\t0.023\t56.168\t0.394\t-0.236\t0.000637\t0.010779\t-3.955\t-0.752\t-0.366\t61.889\t41.490\t-0.404\t98.880\t6\n3170.00\t0.793\t-0.493\t0.000292\t-112.852\t0.023\t56.519\t0.392\t-0.104\t0.000743\t0.012519\t4.124\t-0.895\t-0.378\t62.091\t41.081\t-0.173\t98.430\t6\n3160.00\t0.790\t0.554\t0.000325\t-119.740\t0.023\t56.107\t0.393\t-0.005\t0.000826\t0.013945\t6.874\t-0.940\t-0.537\t61.884\t41.578\t-0.010\t98.652\t6\n3150.00\t0.788\t0.625\t0.000309\t-125.239\t0.024\t56.640\t0.393\t-0.082\t0.000787\t0.013104\t16.637\t-0.842\t-0.595\t62.908\t41.433\t-0.139\t98.588\t6\n3140.00\t0.785\t-0.232\t0.000299\t-125.744\t0.024\t56.475\t0.391\t-0.148\t0.000764\t0.012670\t-7.649\t-0.809\t-0.583\t62.748\t41.583\t-0.255\t98.233\t6\n3130.00\t0.783\t-0.311\t0.000269\t-131.160\t0.023\t55.459\t0.390\t-0.192\t0.000689\t0.011549\t-19.021\t-0.675\t-0.590\t61.609\t42.392\t-0.330\t97.945\t6\n3120.00\t0.780\t0.346\t0.000231\t-131.342\t0.023\t56.492\t0.389\t-0.494\t0.000594\t0.010053\t-5.460\t-0.578\t-0.508\t61.514\t40.742\t-0.840\t97.606\t6\n3110.00\t0.777\t0.392\t0.000210\t-123.761\t0.023\t56.618\t0.387\t-0.538\t0.000542\t0.009127\t-0.003\t-0.581\t-0.389\t61.385\t40.459\t-0.911\t97.019\t6\n3100.00\t0.775\t0.763\t0.000220\t-112.264\t0.023\t55.432\t0.384\t-0.549\t0.000573\t0.009595\t5.963\t-0.680\t-0.279\t60.794\t41.881\t-0.925\t96.469\t6\n3090.00\t0.772\t0.735\t0.000254\t-110.621\t0.023\t56.585\t0.384\t-0.308\t0.000663\t0.011224\t20.849\t-0.793\t-0.298\t60.442\t39.895\t-0.514\t96.215\t6\n3080.00\t0.770\t0.230\t0.000282\t-110.973\t0.023\t56.530\t0.382\t-0.439\t0.000738\t0.012278\t15.152\t-0.878\t-0.337\t61.558\t40.710\t-0.737\t95.898\t6\n3070.00\t0.767\t-0.137\t0.000268\t-118.350\t0.023\t56.750\t0.382\t-0.401\t0.000702\t0.011656\t-5.301\t-0.785\t-0.424\t61.609\t40.405\t-0.671\t95.664\t6\n3060.00\t0.765\t0.137\t0.000257\t-118.273\t0.023\t56.832\t0.379\t-0.275\t0.000678\t0.011358\t-22.312\t-0.755\t-0.406\t61.019\t39.896\t-0.454\t95.239\t6\n3050.00\t0.762\t-0.569\t0.000282\t-116.169\t0.023\t56.992\t0.379\t-0.198\t0.000746\t0.012121\t-44.656\t-0.844\t-0.415\t62.114\t40.368\t-0.322\t94.972\t6\n3040.00\t0.760\t0.621\t0.000277\t-114.401\t0.023\t58.288\t0.377\t-0.313\t0.000736\t0.012074\t-23.445\t-0.842\t-0.382\t62.755\t38.777\t-0.519\t94.626\t6\n3030.00\t0.757\t0.049\t0.000271\t-111.346\t0.023\t57.277\t0.376\t-0.302\t0.000721\t0.011948\t-3.024\t-0.841\t-0.329\t60.923\t39.155\t-0.496\t94.169\t6\n3020.00\t0.755\t0.000\t0.000282\t-113.044\t0.023\t56.212\t0.375\t-0.341\t0.000752\t0.012109\t22.077\t-0.865\t-0.368\t61.695\t41.291\t-0.553\t93.963\t6\n3010.00\t0.752\t-0.382\t0.000291\t-113.170\t0.023\t58.469\t0.374\t-0.269\t0.000779\t0.012853\t34.633\t-0.892\t-0.382\t61.973\t38.029\t-0.437\t93.740\t6\n3000.00\t0.750\t0.731\t0.000296\t-116.559\t0.022\t56.849\t0.372\t-0.148\t0.000796\t0.013246\t17.675\t-0.882\t-0.441\t60.146\t39.299\t-0.245\t93.337\t6\n2990.00\t0.748\t0.209\t0.000299\t-116.060\t0.023\t57.667\t0.371\t-0.324\t0.000805\t0.013003\t-25.314\t-0.894\t-0.437\t61.908\t39.184\t-0.527\t93.180\t6\n2980.00\t0.745\t0.531\t0.000301\t-120.394\t0.023\t57.036\t0.371\t-0.176\t0.000809\t0.013081\t11.996\t-0.864\t-0.507\t62.008\t40.225\t-0.283\t93.088\t6\n2970.00\t0.743\t0.673\t0.000307\t-121.646\t0.023\t58.387\t0.370\t-0.225\t0.000828\t0.013172\t2.509\t-0.871\t-0.536\t63.185\t38.891\t-0.365\t92.932\t6\n2960.00\t0.740\t-0.527\t0.000285\t-118.026\t0.023\t58.019\t0.368\t-0.374\t0.000774\t0.012577\t-17.264\t-0.839\t-0.446\t61.088\t38.133\t-0.599\t92.403\t6\n2950.00\t0.738\t-0.724\t0.000297\t-119.015\t0.023\t58.376\t0.367\t-0.357\t0.000809\t0.013103\t-17.878\t-0.866\t-0.480\t61.823\t38.069\t-0.575\t92.016\t6\n2940.00\t0.735\t0.000\t0.000309\t-122.086\t0.023\t57.453\t0.366\t-0.258\t0.000845\t0.013462\t3.811\t-0.874\t-0.547\t61.683\t39.371\t-0.409\t91.817\t6\n2930.00\t0.733\t0.263\t0.000286\t-120.284\t0.023\t57.777\t0.364\t-0.302\t0.000786\t0.012453\t6.618\t-0.824\t-0.481\t62.286\t39.252\t-0.478\t91.406\t6\n2920.00\t0.730\t0.000\t0.000302\t-123.316\t0.023\t57.942\t0.364\t-0.181\t0.000829\t0.012966\t19.591\t-0.841\t-0.553\t63.225\t39.584\t-0.284\t91.257\t6\n2910.00\t0.728\t0.367\t0.000294\t-121.091\t0.023\t58.348\t0.362\t-0.390\t0.000810\t0.012780\t8.430\t-0.838\t-0.505\t62.295\t38.399\t-0.614\t90.819\t6\n2900.00\t0.725\t0.000\t0.000280\t-123.283\t0.023\t57.958\t0.361\t-0.417\t0.000775\t0.012028\t-18.299\t-0.780\t-0.512\t63.166\t39.523\t-0.657\t90.634\t6\n2890.00\t0.723\t0.000\t0.000284\t-123.964\t0.023\t58.678\t0.360\t-0.170\t0.000790\t0.012547\t-6.975\t-0.786\t-0.529\t62.292\t37.913\t-0.267\t90.371\t6\n2880.00\t0.720\t0.193\t0.000270\t-120.427\t0.023\t58.909\t0.358\t-0.368\t0.000755\t0.011768\t-13.496\t-0.777\t-0.457\t63.257\t38.162\t-0.576\t89.900\t6\n2870.00\t0.717\t-0.674\t0.000273\t-116.356\t0.023\t59.150\t0.356\t-0.357\t0.000765\t0.012034\t-2.543\t-0.814\t-0.404\t61.978\t37.036\t-0.558\t89.359\t6\n2860.00\t0.715\t-0.549\t0.000277\t-113.725\t0.023\t58.777\t0.355\t-0.434\t0.000779\t0.012045\t3.639\t-0.844\t-0.371\t62.543\t37.919\t-0.677\t89.042\t6\n2850.00\t0.712\t-0.518\t0.000307\t-117.806\t0.023\t58.579\t0.355\t-0.121\t0.000865\t0.013181\t17.394\t-0.905\t-0.477\t63.379\t38.722\t-0.183\t89.057\t6\n2840.00\t0.710\t0.690\t0.000298\t-115.763\t0.023\t58.530\t0.354\t-0.302\t0.000844\t0.012992\t10.072\t-0.896\t-0.433\t62.615\t38.331\t-0.470\t88.657\t6\n2830.00\t0.707\t0.273\t0.000333\t-112.621\t0.023\t59.656\t0.351\t-0.236\t0.000949\t0.014494\t-2.397\t-1.024\t-0.427\t63.776\t37.347\t-0.364\t87.970\t6\n2820.00\t0.705\t0.465\t0.000355\t-118.581\t0.023\t58.958\t0.353\t0.126\t0.001008\t0.015473\t22.045\t-1.040\t-0.567\t62.963\t37.907\t0.192\t88.495\t6\n2810.00\t0.702\t0.169\t0.000355\t-120.031\t0.023\t59.914\t0.351\t-0.082\t0.001013\t0.015684\t13.495\t-1.026\t-0.593\t62.385\t36.151\t-0.122\t88.013\t6\n2800.00\t0.700\t0.380\t0.000351\t-128.589\t0.023\t59.573\t0.353\t-0.055\t0.000992\t0.015055\t1.481\t-0.913\t-0.729\t64.115\t37.667\t-0.080\t88.619\t6\n2790.00\t0.697\t-0.397\t0.000339\t-128.870\t0.023\t60.309\t0.352\t-0.187\t0.000965\t0.014576\t5.941\t-0.881\t-0.710\t64.764\t36.924\t-0.282\t88.159\t6\n2780.00\t0.695\t-0.226\t0.000314\t-129.474\t0.023\t58.997\t0.350\t-0.610\t0.000898\t0.013669\t-0.260\t-0.808\t-0.665\t62.722\t37.708\t-0.936\t87.781\t6\n2770.00\t0.692\t-0.637\t0.000317\t-127.057\t0.023\t59.304\t0.346\t-0.637\t0.000915\t0.013793\t3.919\t-0.843\t-0.636\t63.295\t37.590\t-0.968\t86.906\t6\n2760.00\t0.690\t0.564\t0.000323\t-127.062\t0.023\t59.689\t0.346\t-0.396\t0.000936\t0.014073\t-12.032\t-0.860\t-0.649\t63.316\t37.024\t-0.600\t86.628\t6\n2750.00\t0.687\t0.664\t0.000319\t-125.305\t0.023\t59.744\t0.344\t-0.527\t0.000930\t0.013906\t-14.154\t-0.869\t-0.616\t63.183\t36.869\t-0.796\t86.182\t6\n2740.00\t0.685\t-0.312\t0.000304\t-124.882\t0.023\t60.996\t0.343\t-0.500\t0.000887\t0.013244\t5.424\t-0.832\t-0.580\t64.308\t35.652\t-0.745\t85.996\t6\n2730.00\t0.683\t-0.642\t0.000326\t-125.184\t0.023\t59.216\t0.341\t-0.533\t0.000954\t0.014370\t-0.667\t-0.887\t-0.625\t62.047\t36.978\t-0.793\t85.600\t6\n2720.00\t0.680\t0.000\t0.000312\t-125.239\t0.023\t58.749\t0.340\t-0.681\t0.000920\t0.013599\t9.201\t-0.850\t-0.601\t63.074\t38.286\t-1.015\t85.132\t6\n2710.00\t0.678\t0.344\t0.000317\t-124.124\t0.023\t58.524\t0.338\t-0.571\t0.000938\t0.013593\t25.829\t-0.874\t-0.592\t63.401\t38.822\t-0.841\t84.686\t6\n2700.00\t0.675\t0.174\t0.000310\t-124.019\t0.023\t60.084\t0.337\t-0.549\t0.000918\t0.013666\t4.206\t-0.856\t-0.577\t62.962\t36.234\t-0.814\t84.615\t6\n2690.00\t0.673\t-0.224\t0.000318\t-122.959\t0.023\t60.386\t0.335\t-0.670\t0.000949\t0.013822\t0.218\t-0.888\t-0.576\t63.494\t36.083\t-0.980\t83.989\t6\n2680.00\t0.670\t0.450\t0.000345\t-124.612\t0.023\t59.716\t0.334\t-0.527\t0.001034\t0.015233\t-15.664\t-0.947\t-0.653\t62.391\t36.449\t-0.767\t83.681\t6\n2670.00\t0.668\t0.431\t0.000338\t-122.547\t0.023\t59.551\t0.333\t-0.527\t0.001018\t0.014937\t-29.389\t-0.951\t-0.607\t62.312\t36.643\t-0.769\t83.437\t6\n2660.00\t0.665\t-0.181\t0.000342\t-122.591\t0.022\t59.683\t0.331\t-0.511\t0.001033\t0.015315\t15.104\t-0.961\t-0.615\t61.517\t35.987\t-0.740\t83.093\t6\n2650.00\t0.663\t0.621\t0.000358\t-123.948\t0.023\t59.672\t0.330\t-0.577\t0.001084\t0.015801\t1.806\t-0.990\t-0.666\t62.592\t36.625\t-0.835\t82.814\t6\n2640.00\t0.660\t-0.578\t0.000364\t-125.942\t0.023\t60.853\t0.330\t-0.555\t0.001105\t0.016068\t11.378\t-0.983\t-0.712\t63.383\t35.343\t-0.797\t82.705\t6\n2630.00\t0.658\t-0.653\t0.000382\t-126.705\t0.023\t59.941\t0.328\t-0.588\t0.001166\t0.016859\t-2.604\t-1.021\t-0.761\t62.819\t36.365\t-0.842\t82.215\t6\n2620.00\t0.655\t0.365\t0.000378\t-129.293\t0.023\t61.392\t0.326\t-0.720\t0.001159\t0.016467\t-8.603\t-0.976\t-0.798\t64.841\t35.376\t-1.029\t81.864\t6\n2610.00\t0.652\t0.000\t0.000405\t-133.176\t0.022\t59.886\t0.326\t-0.560\t0.001243\t0.018123\t-23.599\t-0.984\t-0.923\t61.899\t35.912\t-0.800\t81.742\t6\n2600.00\t0.650\t0.000\t0.000385\t-138.115\t0.023\t60.601\t0.325\t-0.720\t0.001185\t0.016779\t2.826\t-0.858\t-0.957\t63.879\t35.980\t-1.025\t81.623\t6\n2590.00\t0.647\t-0.631\t0.000393\t-140.707\t0.023\t61.831\t0.323\t-0.637\t0.001218\t0.017116\t8.964\t-0.830\t-1.014\t64.492\t34.548\t-0.898\t80.997\t6\n2580.00\t0.645\t0.000\t0.000366\t-145.602\t0.023\t60.535\t0.322\t-0.747\t0.001138\t0.015951\t15.935\t-0.690\t-1.008\t63.638\t35.946\t-1.048\t80.714\t6\n2570.00\t0.642\t0.624\t0.000318\t-151.567\t0.022\t61.089\t0.321\t-0.577\t0.000989\t0.014223\t41.925\t-0.504\t-0.932\t62.442\t34.484\t-0.810\t80.484\t6\n2560.00\t0.640\t0.000\t0.000339\t-147.887\t0.023\t61.859\t0.320\t-0.659\t0.001061\t0.014753\t28.425\t-0.600\t-0.957\t64.709\t34.622\t-0.922\t80.154\t6\n2550.00\t0.637\t0.000\t0.000286\t-151.100\t0.022\t61.661\t0.318\t-0.775\t0.000901\t0.013004\t7.677\t-0.462\t-0.836\t62.334\t33.628\t-1.076\t79.700\t6\n2540.00\t0.635\t0.382\t0.000262\t-150.639\t0.022\t61.100\t0.316\t-0.851\t0.000830\t0.011905\t-15.938\t-0.429\t-0.762\t61.873\t34.155\t-1.175\t79.278\t6\n2530.00\t0.632\t0.357\t0.000255\t-146.805\t0.022\t61.452\t0.313\t-1.066\t0.000814\t0.011401\t-39.983\t-0.465\t-0.710\t62.504\t34.013\t-1.458\t78.518\t6\n2520.00\t0.630\t0.000\t0.000263\t-133.720\t0.023\t61.100\t0.317\t-1.000\t0.000829\t0.011588\t-24.739\t-0.632\t-0.605\t63.304\t34.946\t-1.385\t79.429\t6\n2510.00\t0.627\t-0.219\t0.000265\t-142.723\t0.022\t61.155\t0.309\t-0.934\t0.000857\t0.011870\t-6.916\t-0.535\t-0.703\t62.445\t34.400\t-1.269\t77.612\t6\n2500.00\t0.625\t-0.625\t0.000200\t-133.687\t0.022\t61.837\t0.311\t-0.687\t0.000643\t0.008960\t-20.098\t-0.483\t-0.461\t63.371\t33.938\t-0.938\t78.123\t6\n2490.00\t0.623\t-0.619\t0.000243\t-136.055\t0.022\t61.392\t0.310\t-0.676\t0.000785\t0.010891\t13.023\t-0.563\t-0.584\t62.576\t34.134\t-0.919\t77.739\t6\n2480.00\t0.620\t-0.363\t0.000261\t-137.351\t0.023\t62.172\t0.309\t-0.698\t0.000847\t0.011539\t11.782\t-0.591\t-0.641\t63.961\t33.774\t-0.942\t77.451\t6\n2470.00\t0.618\t-0.247\t0.000243\t-132.979\t0.022\t62.078\t0.307\t-0.780\t0.000793\t0.011047\t23.020\t-0.593\t-0.553\t62.722\t33.256\t-1.046\t76.998\t6\n2460.00\t0.615\t0.558\t0.000244\t-134.572\t0.022\t60.947\t0.306\t-0.851\t0.000798\t0.010932\t17.091\t-0.580\t-0.571\t62.529\t34.734\t-1.143\t76.773\t6\n2450.00\t0.613\t0.000\t0.000252\t-132.676\t0.022\t61.891\t0.305\t-0.731\t0.000825\t0.011269\t19.368\t-0.617\t-0.569\t63.362\t33.859\t-0.976\t76.525\t6\n2440.00\t0.610\t-0.488\t0.000252\t-131.951\t0.022\t62.776\t0.303\t-0.780\t0.000830\t0.011275\t16.929\t-0.625\t-0.561\t63.483\t32.663\t-1.033\t76.061\t6\n2430.00\t0.608\t0.537\t0.000260\t-125.678\t0.022\t61.990\t0.302\t-0.736\t0.000863\t0.011646\t13.077\t-0.704\t-0.506\t63.131\t33.594\t-0.973\t75.704\t6\n2420.00\t0.605\t0.000\t0.000249\t-127.189\t0.022\t61.968\t0.300\t-0.857\t0.000829\t0.011299\t-19.570\t-0.661\t-0.501\t62.495\t33.291\t-1.126\t75.299\t6\n2410.00\t0.603\t-0.603\t0.000259\t-124.656\t0.022\t62.161\t0.299\t-0.890\t0.000865\t0.011737\t-21.311\t-0.709\t-0.490\t61.899\t32.699\t-1.162\t74.975\t6\n2400.00\t0.600\t0.000\t0.000276\t-131.342\t0.022\t62.023\t0.299\t-0.687\t0.000924\t0.012348\t-12.706\t-0.690\t-0.608\t62.822\t33.380\t-0.900\t74.966\t6\n2390.00\t0.598\t0.581\t0.000258\t-130.792\t0.022\t62.062\t0.298\t-0.829\t0.000865\t0.011528\t-5.371\t-0.650\t-0.561\t63.432\t33.652\t-1.077\t74.618\t6\n2380.00\t0.595\t0.000\t0.000259\t-128.760\t0.022\t62.825\t0.295\t-0.725\t0.000879\t0.011779\t7.062\t-0.674\t-0.541\t63.134\t32.416\t-0.934\t74.085\t6\n2370.00\t0.592\t0.000\t0.000271\t-126.832\t0.022\t61.897\t0.294\t-0.797\t0.000922\t0.012118\t7.724\t-0.722\t-0.541\t62.694\t33.490\t-1.022\t73.685\t6\n2360.00\t0.590\t-0.437\t0.000253\t-133.369\t0.022\t62.100\t0.294\t-0.846\t0.000861\t0.011331\t2.341\t-0.613\t-0.579\t63.111\t33.426\t-1.090\t73.740\t6\n2350.00\t0.587\t-0.072\t0.000260\t-131.353\t0.022\t62.919\t0.293\t-0.824\t0.000888\t0.011625\t5.697\t-0.650\t-0.572\t63.303\t32.368\t-1.058\t73.379\t6\n2340.00\t0.585\t0.515\t0.000261\t-127.645\t0.022\t62.172\t0.290\t-0.813\t0.000901\t0.011693\t5.412\t-0.689\t-0.532\t63.431\t33.495\t-1.033\t72.787\t6\n2330.00\t0.582\t0.517\t0.000259\t-131.869\t0.022\t63.045\t0.290\t-0.829\t0.000894\t0.011751\t4.554\t-0.642\t-0.576\t62.500\t31.781\t-1.054\t72.620\t6\n2320.00\t0.580\t-0.579\t0.000261\t-129.924\t0.022\t62.924\t0.288\t-0.912\t0.000905\t0.011828\t22.137\t-0.666\t-0.557\t63.209\t32.314\t-1.150\t72.254\t6\n2310.00\t0.577\t0.336\t0.000284\t-127.123\t0.022\t62.952\t0.286\t-0.698\t0.000994\t0.012895\t4.125\t-0.755\t-0.571\t62.541\t31.935\t-0.873\t71.668\t6\n2300.00\t0.575\t0.335\t0.000277\t-128.013\t0.022\t63.995\t0.284\t-0.879\t0.000972\t0.012558\t-2.556\t-0.726\t-0.568\t62.917\t30.699\t-1.094\t71.319\t6\n2290.00\t0.572\t0.196\t0.000266\t-127.447\t0.022\t62.979\t0.283\t-0.764\t0.000940\t0.012059\t-4.120\t-0.703\t-0.538\t62.652\t31.953\t-0.945\t70.957\t6\n2280.00\t0.570\t-0.085\t0.000259\t-127.414\t0.022\t62.556\t0.282\t-1.077\t0.000918\t0.011754\t-2.957\t-0.685\t-0.524\t62.371\t32.396\t-1.332\t70.799\t6\n2270.00\t0.567\t-0.441\t0.000281\t-130.232\t0.022\t63.809\t0.281\t-0.846\t0.000999\t0.012764\t-8.192\t-0.716\t-0.605\t63.563\t31.266\t-1.042\t70.576\t6\n2260.00\t0.565\t0.330\t0.000244\t-134.550\t0.022\t62.199\t0.282\t-1.719\t0.000864\t0.011055\t10.580\t-0.578\t-0.569\t62.530\t32.983\t-2.126\t70.677\t6\n2250.00\t0.562\t0.199\t0.000279\t-124.651\t0.022\t63.517\t0.277\t-1.055\t0.001007\t0.012830\t6.737\t-0.764\t-0.528\t62.090\t30.923\t-1.279\t69.396\t6\n2240.00\t0.560\t-0.421\t0.000273\t-130.287\t0.022\t64.303\t0.278\t-0.829\t0.000983\t0.012391\t7.979\t-0.694\t-0.588\t63.694\t30.662\t-1.007\t69.621\t6\n2230.00\t0.558\t-0.558\t0.000295\t-128.282\t0.022\t64.072\t0.275\t-0.522\t0.001074\t0.013589\t-1.729\t-0.772\t-0.609\t62.087\t30.192\t-0.627\t68.900\t6\n2220.00\t0.555\t-0.054\t0.000304\t-132.737\t0.022\t64.627\t0.275\t-0.203\t0.001103\t0.013785\t16.039\t-0.743\t-0.687\t63.685\t30.214\t-0.246\t68.981\t6\n2210.00\t0.553\t0.338\t0.000286\t-135.082\t0.022\t63.962\t0.274\t-0.577\t0.001045\t0.012816\t3.250\t-0.674\t-0.676\t63.959\t31.247\t-0.691\t68.726\t6\n2200.00\t0.550\t0.366\t0.000267\t-135.577\t0.022\t63.693\t0.273\t-0.868\t0.000977\t0.012119\t-12.214\t-0.623\t-0.635\t63.322\t31.302\t-1.038\t68.581\t6\n2190.00\t0.548\t-0.420\t0.000254\t-131.616\t0.022\t63.869\t0.271\t-0.956\t0.000935\t0.011513\t-7.115\t-0.632\t-0.561\t63.080\t30.946\t-1.135\t68.072\t6\n2180.00\t0.545\t0.220\t0.000268\t-133.726\t0.022\t63.907\t0.270\t-0.747\t0.000990\t0.012331\t-5.998\t-0.645\t-0.617\t62.820\t30.769\t-0.885\t67.850\t6\n2170.00\t0.543\t0.524\t0.000264\t-132.764\t0.022\t64.935\t0.269\t-0.934\t0.000983\t0.011993\t5.128\t-0.646\t-0.598\t64.121\t29.997\t-1.102\t67.425\t6\n2160.00\t0.540\t0.201\t0.000281\t-128.886\t0.022\t64.814\t0.267\t-0.692\t0.001053\t0.012745\t10.041\t-0.729\t-0.587\t64.009\t30.116\t-0.810\t66.902\t6\n2150.00\t0.538\t-0.082\t0.000294\t-133.506\t0.022\t64.479\t0.266\t-0.461\t0.001102\t0.013525\t20.408\t-0.710\t-0.674\t62.653\t29.919\t-0.541\t66.868\t6\n2140.00\t0.535\t-0.408\t0.000276\t-134.132\t0.022\t64.622\t0.266\t-0.665\t0.001037\t0.012524\t9.400\t-0.660\t-0.640\t63.852\t30.297\t-0.772\t66.751\t6\n2130.00\t0.533\t-0.461\t0.000280\t-132.808\t0.022\t64.913\t0.264\t-0.648\t0.001062\t0.012546\t6.686\t-0.685\t-0.635\t64.331\t30.131\t-0.750\t66.226\t6\n2120.00\t0.530\t0.000\t0.000270\t-130.825\t0.022\t64.490\t0.262\t-0.829\t0.001031\t0.012238\t-6.591\t-0.680\t-0.587\t63.198\t30.170\t-0.952\t65.635\t6\n2110.00\t0.527\t0.283\t0.000274\t-132.490\t0.022\t65.720\t0.261\t-0.665\t0.001050\t0.012629\t-8.040\t-0.674\t-0.617\t63.359\t28.586\t-0.758\t65.540\t6\n2100.00\t0.525\t-0.405\t0.000257\t-130.380\t0.022\t64.973\t0.260\t-0.862\t0.000990\t0.011844\t-26.721\t-0.653\t-0.555\t62.914\t29.382\t-0.978\t65.150\t6\n2090.00\t0.522\t-0.080\t0.000271\t-131.605\t0.022\t64.446\t0.259\t-0.890\t0.001047\t0.012462\t-22.512\t-0.674\t-0.599\t62.951\t30.110\t-1.006\t64.856\t6\n2080.00\t0.520\t-0.007\t0.000258\t-131.951\t0.022\t65.220\t0.257\t-0.797\t0.001002\t0.011881\t7.096\t-0.639\t-0.575\t63.245\t29.203\t-0.897\t64.570\t6\n2070.00\t0.517\t0.450\t0.000261\t-130.452\t0.022\t65.753\t0.257\t-0.857\t0.001017\t0.011857\t1.096\t-0.662\t-0.565\t64.001\t28.832\t-0.966\t64.390\t6\n2060.00\t0.515\t0.240\t0.000268\t-131.682\t0.022\t63.336\t0.255\t-0.709\t0.001050\t0.012153\t0.193\t-0.666\t-0.593\t62.850\t31.553\t-0.793\t63.984\t6\n2050.00\t0.512\t-0.397\t0.000273\t-132.995\t0.022\t65.737\t0.255\t-0.670\t0.001071\t0.012551\t17.794\t-0.664\t-0.620\t63.419\t28.586\t-0.750\t63.876\t6\n2040.00\t0.510\t-0.499\t0.000256\t-130.265\t0.022\t66.171\t0.252\t-0.846\t0.001015\t0.011797\t4.625\t-0.651\t-0.552\t63.908\t28.217\t-0.933\t63.277\t6\n2030.00\t0.507\t0.460\t0.000270\t-129.611\t0.022\t65.814\t0.251\t-0.665\t0.001076\t0.012259\t2.172\t-0.693\t-0.574\t64.020\t28.759\t-0.729\t62.987\t6\n2020.00\t0.505\t0.000\t0.000275\t-131.457\t0.022\t66.522\t0.250\t-0.582\t0.001100\t0.012465\t18.108\t-0.686\t-0.606\t64.692\t28.093\t-0.637\t62.631\t6\n2010.00\t0.502\t0.000\t0.000265\t-131.622\t0.022\t66.434\t0.248\t-0.797\t0.001066\t0.012188\t11.836\t-0.659\t-0.586\t63.731\t27.788\t-0.866\t62.303\t6\n2000.00\t0.500\t-0.359\t0.000284\t-129.018\t0.021\t66.220\t0.247\t-0.901\t0.001147\t0.013251\t6.883\t-0.734\t-0.595\t63.063\t27.783\t-0.975\t62.012\t6\n1990.00\t0.498\t0.300\t0.000266\t-130.831\t0.022\t65.912\t0.247\t-0.818\t0.001075\t0.012234\t-19.055\t-0.670\t-0.579\t63.558\t28.416\t-0.885\t62.019\t6\n1980.00\t0.495\t0.000\t0.000266\t-127.722\t0.022\t65.945\t0.245\t-0.742\t0.001086\t0.012061\t-12.666\t-0.700\t-0.542\t64.447\t28.765\t-0.795\t61.411\t6\n1970.00\t0.493\t0.431\t0.000281\t-132.638\t0.021\t65.940\t0.243\t-0.923\t0.001158\t0.013120\t-6.495\t-0.688\t-0.634\t62.394\t27.861\t-0.981\t60.868\t6\n1960.00\t0.490\t-0.489\t0.000255\t-134.138\t0.022\t64.111\t0.242\t-0.286\t0.001056\t0.011432\t-16.344\t-0.611\t-0.593\t64.290\t31.204\t-0.300\t60.602\t6\n1950.00\t0.488\t-0.036\t0.000241\t-134.088\t0.022\t66.072\t0.240\t-0.544\t0.001005\t0.011118\t-15.284\t-0.578\t-0.560\t63.730\t28.272\t-0.569\t60.230\t6\n1940.00\t0.485\t-0.423\t0.000257\t-131.770\t0.022\t64.995\t0.240\t-0.604\t0.001070\t0.011487\t-1.056\t-0.638\t-0.570\t64.385\t30.039\t-0.635\t60.185\t6\n1930.00\t0.482\t0.252\t0.000268\t-130.177\t0.021\t65.731\t0.239\t-0.835\t0.001124\t0.012524\t22.633\t-0.682\t-0.576\t62.835\t28.332\t-0.873\t59.852\t6\n1920.00\t0.480\t0.410\t0.000277\t-131.852\t0.022\t65.995\t0.237\t-0.615\t0.001168\t0.012753\t-3.598\t-0.687\t-0.616\t63.510\t28.282\t-0.637\t59.490\t6\n1910.00\t0.477\t0.453\t0.000276\t-134.918\t0.022\t65.424\t0.237\t-0.670\t0.001164\t0.012700\t-4.199\t-0.651\t-0.649\t63.290\t28.954\t-0.698\t59.460\t6\n1900.00\t0.475\t0.028\t0.000265\t-130.792\t0.021\t67.593\t0.234\t-0.829\t0.001130\t0.012369\t10.075\t-0.668\t-0.576\t63.343\t26.127\t-0.850\t58.803\t6\n1890.00\t0.472\t0.451\t0.000263\t-134.044\t0.022\t66.313\t0.233\t-0.736\t0.001127\t0.012100\t6.472\t-0.629\t-0.609\t63.199\t27.717\t-0.751\t58.465\t6\n1880.00\t0.470\t0.000\t0.000262\t-130.589\t0.022\t67.928\t0.232\t-0.840\t0.001130\t0.012081\t0.100\t-0.664\t-0.569\t63.951\t25.943\t-0.853\t58.246\t6\n1870.00\t0.468\t-0.374\t0.000266\t-135.297\t0.021\t66.731\t0.231\t-0.786\t0.001149\t0.012611\t-3.705\t-0.624\t-0.630\t62.081\t26.697\t-0.799\t58.062\t6\n1860.00\t0.465\t0.231\t0.000267\t-132.764\t0.022\t65.297\t0.230\t-1.000\t0.001159\t0.012113\t12.824\t-0.653\t-0.604\t63.708\t29.315\t-1.006\t57.740\t6\n1850.00\t0.463\t0.457\t0.000262\t-134.022\t0.021\t66.918\t0.229\t-0.714\t0.001147\t0.012437\t24.218\t-0.628\t-0.608\t61.657\t26.275\t-0.713\t57.349\t6\n1840.00\t0.460\t-0.016\t0.000255\t-129.452\t0.021\t67.214\t0.227\t-0.939\t0.001124\t0.011901\t12.676\t-0.655\t-0.539\t63.004\t26.474\t-0.933\t56.844\t6\n1830.00\t0.458\t-0.455\t0.000267\t-137.653\t0.021\t66.368\t0.226\t-0.895\t0.001181\t0.012463\t-11.211\t-0.599\t-0.657\t62.449\t27.310\t-0.887\t56.681\t6\n1820.00\t0.455\t-0.322\t0.000268\t-131.770\t0.022\t67.061\t0.225\t-0.884\t0.001188\t0.012338\t-42.163\t-0.666\t-0.595\t63.737\t26.979\t-0.873\t56.487\t6\n1810.00\t0.452\t0.000\t0.000271\t-134.940\t0.022\t67.775\t0.224\t-0.840\t0.001210\t0.012460\t-15.988\t-0.638\t-0.637\t64.438\t26.340\t-0.820\t56.082\t6\n1800.00\t0.450\t0.289\t0.000247\t-128.463\t0.021\t67.407\t0.221\t-0.884\t0.001119\t0.011721\t14.389\t-0.645\t-0.512\t62.358\t25.956\t-0.856\t55.411\t6\n1790.00\t0.447\t-0.083\t0.000251\t-129.672\t0.021\t67.786\t0.220\t-0.615\t0.001141\t0.011923\t5.967\t-0.645\t-0.535\t62.292\t25.447\t-0.591\t55.292\t6\n1780.00\t0.445\t0.000\t0.000240\t-120.630\t0.021\t68.829\t0.219\t-0.698\t0.001096\t0.011549\t10.849\t-0.688\t-0.408\t62.423\t24.174\t-0.667\t54.882\t6\n1770.00\t0.442\t-0.025\t0.000279\t-129.260\t0.022\t68.637\t0.219\t-0.571\t0.001275\t0.012837\t10.840\t-0.719\t-0.588\t64.279\t25.146\t-0.546\t54.854\t6\n1760.00\t0.440\t0.403\t0.000250\t-127.831\t0.021\t68.176\t0.217\t-0.736\t0.001154\t0.011689\t21.644\t-0.658\t-0.511\t63.673\t25.510\t-0.700\t54.411\t6\n1750.00\t0.437\t-0.007\t0.000278\t-128.199\t0.021\t67.269\t0.215\t-0.934\t0.001291\t0.012987\t18.475\t-0.728\t-0.573\t63.580\t26.643\t-0.882\t53.971\t6\n1740.00\t0.435\t0.000\t0.000278\t-132.545\t0.022\t67.110\t0.216\t-0.632\t0.001289\t0.012809\t-17.722\t-0.683\t-0.627\t63.739\t26.916\t-0.596\t54.152\t6\n1730.00\t0.433\t0.000\t0.000254\t-125.925\t0.022\t68.483\t0.213\t-1.066\t0.001190\t0.011688\t-21.427\t-0.685\t-0.496\t64.365\t25.380\t-0.993\t53.475\t6\n1720.00\t0.430\t0.182\t0.000265\t-126.277\t0.021\t67.011\t0.210\t-1.280\t0.001262\t0.012575\t7.272\t-0.712\t-0.523\t62.501\t26.519\t-1.175\t52.689\t6\n1710.00\t0.428\t0.000\t0.000246\t-140.691\t0.021\t66.259\t0.211\t-1.247\t0.001164\t0.011667\t3.299\t-0.519\t-0.634\t61.625\t27.095\t-1.155\t53.007\t6\n1700.00\t0.425\t-0.283\t0.000163\t-111.539\t0.020\t69.818\t0.203\t-1.747\t0.000804\t0.008111\t9.484\t-0.506\t-0.200\t60.414\t22.203\t-1.556\t50.931\t6\n1690.00\t0.423\t-0.422\t0.000298\t-104.908\t0.020\t68.906\t0.201\t0.352\t0.001486\t0.014592\t-16.556\t-0.961\t-0.256\t60.965\t23.516\t0.312\t50.453\t6\n1680.00\t0.420\t0.000\t0.000332\t-114.357\t0.021\t68.126\t0.202\t0.928\t0.001641\t0.015966\t-15.316\t-1.007\t-0.456\t61.521\t24.709\t0.821\t50.698\t6\n1670.00\t0.417\t0.000\t0.000294\t-128.919\t0.021\t68.000\t0.205\t-0.319\t0.001434\t0.014163\t-2.919\t-0.763\t-0.616\t61.891\t25.016\t-0.285\t51.402\t6\n1660.00\t0.415\t0.209\t0.000293\t-133.467\t0.021\t69.203\t0.206\t-0.148\t0.001426\t0.013909\t0.608\t-0.709\t-0.672\t63.131\t23.970\t-0.133\t51.630\t6\n1650.00\t0.412\t0.000\t0.000254\t-131.858\t0.021\t69.423\t0.202\t-0.775\t0.001258\t0.012055\t-8.771\t-0.631\t-0.565\t63.338\t23.768\t-0.687\t50.698\t6\n1640.00\t0.410\t-0.393\t0.000251\t-132.330\t0.021\t68.066\t0.202\t-0.654\t0.001246\t0.012095\t5.239\t-0.619\t-0.564\t61.502\t24.779\t-0.577\t50.612\t6\n1630.00\t0.407\t0.000\t0.000276\t-129.408\t0.021\t68.269\t0.200\t-0.527\t0.001382\t0.013111\t27.890\t-0.712\t-0.585\t62.743\t25.019\t-0.464\t50.211\t6\n1620.00\t0.405\t0.000\t0.000255\t-129.600\t0.021\t69.500\t0.198\t-0.533\t0.001285\t0.011908\t38.885\t-0.654\t-0.541\t64.106\t23.963\t-0.462\t49.754\t6\n1610.00\t0.403\t-0.081\t0.000271\t-127.095\t0.021\t69.033\t0.197\t-0.401\t0.001372\t0.013028\t7.029\t-0.719\t-0.544\t62.394\t23.910\t-0.348\t49.493\t6\n1600.00\t0.400\t-0.399\t0.000252\t-126.469\t0.021\t70.417\t0.197\t-0.604\t0.001283\t0.012150\t-6.106\t-0.676\t-0.500\t62.897\t22.381\t-0.522\t49.360\t6\n1590.00\t0.398\t-0.390\t0.000264\t-131.836\t0.021\t70.692\t0.196\t-0.681\t0.001348\t0.012325\t7.236\t-0.655\t-0.586\t64.176\t22.491\t-0.584\t49.069\t6\n1580.00\t0.395\t0.071\t0.000281\t-127.068\t0.021\t69.703\t0.194\t-0.242\t0.001449\t0.013539\t0.183\t-0.748\t-0.565\t62.722\t23.195\t-0.204\t48.713\t6\n1570.00\t0.393\t0.357\t0.000279\t-125.645\t0.021\t70.516\t0.192\t-0.159\t0.001453\t0.013429\t-21.869\t-0.755\t-0.542\t63.025\t22.309\t-0.134\t48.180\t6\n1560.00\t0.390\t-0.313\t0.000305\t-129.034\t0.021\t68.560\t0.192\t0.099\t0.001589\t0.014460\t-12.316\t-0.789\t-0.640\t62.400\t24.510\t0.083\t48.132\t6\n1550.00\t0.387\t-0.325\t0.000285\t-133.423\t0.021\t68.632\t0.192\t-0.423\t0.001485\t0.013536\t0.469\t-0.691\t-0.654\t62.782\t24.571\t-0.354\t48.226\t6\n1540.00\t0.385\t0.000\t0.000266\t-128.859\t0.021\t69.500\t0.189\t-0.797\t0.001405\t0.012598\t-4.136\t-0.689\t-0.555\t63.501\t23.733\t-0.659\t47.444\t6\n1530.00\t0.382\t0.170\t0.000280\t-130.556\t0.021\t69.988\t0.188\t-0.472\t0.001484\t0.013259\t-10.744\t-0.708\t-0.606\t63.572\t23.156\t-0.387\t47.270\t6\n1520.00\t0.380\t0.000\t0.000263\t-129.897\t0.020\t70.247\t0.186\t-0.242\t0.001410\t0.013048\t-8.552\t-0.672\t-0.562\t60.743\t21.817\t-0.195\t46.795\t6\n1510.00\t0.377\t-0.376\t0.000283\t-132.742\t0.020\t71.180\t0.186\t-0.236\t0.001525\t0.013829\t-17.364\t-0.692\t-0.640\t62.035\t21.149\t-0.193\t46.567\t6\n1500.00\t0.375\t-0.313\t0.000275\t-133.055\t0.020\t70.411\t0.184\t-0.209\t0.001495\t0.013437\t5.060\t-0.669\t-0.625\t61.698\t21.964\t-0.169\t46.115\t6\n1490.00\t0.373\t0.371\t0.000264\t-124.327\t0.020\t71.400\t0.182\t-0.049\t0.001447\t0.012901\t9.506\t-0.726\t-0.496\t61.802\t20.805\t-0.039\t45.759\t6\n1480.00\t0.370\t0.000\t0.000269\t-127.820\t0.021\t69.928\t0.180\t-0.357\t0.001498\t0.012965\t7.862\t-0.709\t-0.550\t62.420\t22.809\t-0.280\t45.084\t6\n1470.00\t0.368\t0.000\t0.000254\t-124.810\t0.020\t71.746\t0.179\t-0.214\t0.001413\t0.012590\t18.584\t-0.694\t-0.483\t61.618\t20.332\t-0.166\t45.012\t6\n1460.00\t0.365\t-0.305\t0.000272\t-128.386\t0.021\t71.658\t0.180\t-0.154\t0.001514\t0.012708\t16.076\t-0.710\t-0.563\t64.605\t21.424\t-0.121\t45.072\t6\n1450.00\t0.363\t-0.157\t0.000278\t-129.150\t0.021\t70.455\t0.177\t0.115\t0.001575\t0.013408\t4.628\t-0.720\t-0.586\t62.589\t22.229\t0.088\t44.371\t6\n1440.00\t0.360\t0.000\t0.000277\t-123.173\t0.021\t71.900\t0.175\t-0.280\t0.001582\t0.013314\t-15.678\t-0.771\t-0.504\t63.591\t20.792\t-0.215\t43.859\t6\n1430.00\t0.357\t-0.077\t0.000277\t-125.013\t0.020\t72.713\t0.170\t0.967\t0.001628\t0.013758\t-15.808\t-0.756\t-0.530\t61.956\t19.276\t0.721\t42.687\t6\n1420.00\t0.355\t-0.296\t0.000311\t-129.540\t0.020\t76.218\t0.173\t4.828\t0.001793\t0.015204\t-14.112\t-0.799\t-0.660\t63.645\t15.608\t3.665\t43.376\t6\n1410.00\t0.352\t0.064\t0.000255\t-133.660\t0.022\t76.635\t0.182\t4.005\t0.001404\t0.011755\t12.300\t-0.616\t-0.587\t67.473\t16.035\t3.189\t45.533\t6\n1400.00\t0.350\t-0.189\t0.000260\t-132.281\t0.023\t64.385\t0.184\t-4.774\t0.001416\t0.011472\t-3.327\t-0.641\t-0.583\t65.361\t31.344\t-3.837\t45.902\t6\n1390.00\t0.347\t0.023\t0.000259\t-135.330\t0.021\t67.495\t0.171\t-1.967\t0.001514\t0.012460\t39.573\t-0.607\t-0.613\t61.618\t25.538\t-1.472\t42.853\t6\n1380.00\t0.345\t0.119\t0.000266\t-129.446\t0.021\t68.752\t0.173\t-2.010\t0.001544\t0.012821\t9.214\t-0.685\t-0.564\t62.222\t24.200\t-1.516\t43.247\t6\n1370.00\t0.343\t-0.338\t0.000277\t-119.026\t0.021\t71.587\t0.168\t-1.044\t0.001644\t0.013123\t-7.035\t-0.807\t-0.448\t63.996\t21.316\t-0.771\t42.240\t6\n1360.00\t0.340\t0.154\t0.000282\t-125.398\t0.021\t70.719\t0.167\t-1.159\t0.001690\t0.013371\t-6.182\t-0.766\t-0.544\t63.983\t22.394\t-0.847\t41.839\t6\n1350.00\t0.338\t0.000\t0.000277\t-122.789\t0.020\t72.235\t0.165\t-0.242\t0.001684\t0.013565\t-8.018\t-0.777\t-0.501\t62.723\t20.096\t-0.175\t41.387\t6\n1340.00\t0.335\t0.193\t0.000296\t-123.871\t0.021\t72.131\t0.164\t-0.231\t0.001805\t0.014026\t2.179\t-0.818\t-0.549\t64.475\t20.789\t-0.164\t41.126\t6\n1330.00\t0.333\t-0.319\t0.000272\t-123.508\t0.021\t71.686\t0.163\t-0.286\t0.001670\t0.013105\t16.562\t-0.756\t-0.501\t62.660\t20.749\t-0.205\t40.899\t6\n1320.00\t0.330\t-0.082\t0.000308\t-121.465\t0.021\t71.565\t0.161\t-0.549\t0.001908\t0.014596\t0.925\t-0.875\t-0.535\t64.465\t21.500\t-0.387\t40.478\t6\n1310.00\t0.327\t0.000\t0.000292\t-126.744\t0.021\t71.252\t0.161\t-0.038\t0.001814\t0.013627\t2.524\t-0.779\t-0.581\t64.644\t21.948\t-0.025\t40.356\t6\n1300.00\t0.325\t0.000\t0.000283\t-125.903\t0.021\t70.994\t0.159\t-0.489\t0.001780\t0.013438\t-6.929\t-0.765\t-0.554\t63.389\t21.849\t-0.342\t39.933\t6\n1290.00\t0.322\t0.000\t0.000303\t-128.452\t0.021\t70.774\t0.159\t-0.236\t0.001904\t0.014354\t-23.077\t-0.790\t-0.627\t63.814\t22.268\t-0.166\t39.835\t6\n1280.00\t0.320\t-0.314\t0.000293\t-120.569\t0.020\t73.010\t0.157\t-0.110\t0.001869\t0.014343\t7.398\t-0.842\t-0.498\t63.009\t19.250\t-0.075\t39.374\t6\n1270.00\t0.317\t0.244\t0.000329\t-125.557\t0.022\t72.416\t0.156\t-0.033\t0.002112\t0.015166\t39.295\t-0.893\t-0.638\t66.606\t21.102\t-0.021\t39.118\t6\n1260.00\t0.315\t0.230\t0.000300\t-130.820\t0.021\t70.532\t0.155\t-0.560\t0.001936\t0.014428\t27.576\t-0.756\t-0.653\t63.034\t22.292\t-0.381\t38.819\t6\n1250.00\t0.312\t0.120\t0.000259\t-129.133\t0.021\t71.296\t0.155\t-0.352\t0.001677\t0.012474\t18.150\t-0.670\t-0.545\t63.035\t21.351\t-0.238\t38.755\t6\n1240.00\t0.310\t-0.307\t0.000314\t-132.638\t0.021\t71.032\t0.153\t-0.220\t0.002058\t0.014912\t1.685\t-0.771\t-0.710\t64.016\t22.013\t-0.147\t38.352\t6\n1230.00\t0.308\t0.000\t0.000266\t-134.539\t0.020\t70.439\t0.151\t-0.264\t0.001760\t0.012994\t-19.089\t-0.631\t-0.621\t61.843\t21.984\t-0.175\t37.904\t6\n1220.00\t0.305\t0.216\t0.000276\t-114.802\t0.021\t72.499\t0.149\t-0.203\t0.001853\t0.013286\t-18.317\t-0.835\t-0.386\t63.821\t20.118\t-0.132\t37.383\t6\n1210.00\t0.303\t0.000\t0.000274\t-120.619\t0.020\t73.943\t0.148\t0.280\t0.001857\t0.013413\t-7.715\t-0.787\t-0.466\t62.992\t18.137\t0.182\t37.054\t6\n1200.00\t0.300\t0.000\t0.000314\t-124.783\t0.021\t72.394\t0.148\t0.577\t0.002124\t0.014889\t-1.231\t-0.859\t-0.597\t64.661\t20.513\t0.375\t37.094\t6\n1190.00\t0.298\t-0.244\t0.000301\t-122.624\t0.021\t73.806\t0.146\t0.396\t0.002058\t0.014065\t-13.964\t-0.845\t-0.541\t65.666\t19.079\t0.254\t36.715\t6\n1180.00\t0.295\t0.000\t0.000326\t-124.426\t0.021\t73.339\t0.144\t0.000\t0.002261\t0.015252\t-6.502\t-0.897\t-0.615\t65.484\t19.599\t-0.001\t36.233\t6\n1170.00\t0.292\t0.000\t0.000330\t-134.236\t0.021\t71.505\t0.144\t-0.165\t0.002295\t0.015877\t-6.256\t-0.787\t-0.767\t63.168\t21.138\t-0.104\t36.046\t6\n1160.00\t0.290\t-0.106\t0.000269\t-133.868\t0.020\t70.670\t0.141\t-0.236\t0.001907\t0.013591\t-3.898\t-0.647\t-0.623\t60.177\t21.120\t-0.144\t35.441\t6\n1150.00\t0.287\t-0.286\t0.000247\t-125.793\t0.020\t73.279\t0.138\t-0.610\t0.001796\t0.012682\t5.541\t-0.669\t-0.483\t60.209\t18.092\t-0.369\t34.568\t6\n1140.00\t0.285\t0.000\t0.000334\t-103.914\t0.021\t77.783\t0.137\t2.554\t0.002443\t0.015597\t117.049\t-1.080\t-0.268\t67.121\t14.538\t1.528\t34.222\t6\n1130.00\t0.282\t0.000\t0.000303\t-115.977\t0.022\t76.174\t0.140\t2.466\t0.002161\t0.013955\t102.207\t-0.908\t-0.442\t67.593\t16.630\t1.514\t35.140\t6\n1120.00\t0.280\t0.183\t0.000353\t-111.731\t0.022\t74.213\t0.142\t1.631\t0.002484\t0.016264\t-2.291\t-1.093\t-0.436\t66.779\t18.891\t1.015\t35.636\t6\n1110.00\t0.278\t-0.186\t0.000343\t-126.013\t0.021\t73.663\t0.139\t-0.115\t0.002461\t0.016271\t-127.319\t-0.925\t-0.672\t64.475\t18.901\t-0.071\t34.987\t6\n1100.00\t0.275\t-0.224\t0.000327\t-132.539\t0.021\t71.356\t0.135\t-0.824\t0.002417\t0.015752\t-115.121\t-0.803\t-0.737\t63.214\t21.340\t-0.487\t33.977\t6\n1090.00\t0.273\t0.041\t0.000307\t-127.617\t0.020\t73.081\t0.135\t0.560\t0.002282\t0.015261\t-67.531\t-0.811\t-0.625\t62.169\t18.909\t0.331\t33.820\t6\n1080.00\t0.270\t0.252\t0.000297\t-124.563\t0.021\t73.191\t0.132\t-0.148\t0.002251\t0.014310\t7.811\t-0.816\t-0.562\t63.271\t19.117\t-0.086\t33.128\t6\n1070.00\t0.268\t-0.092\t0.000289\t-131.023\t0.020\t73.026\t0.132\t-0.110\t0.002185\t0.014122\t32.931\t-0.726\t-0.632\t62.594\t19.107\t-0.064\t33.144\t6\n1060.00\t0.265\t-0.264\t0.000286\t-124.464\t0.020\t75.388\t0.131\t0.330\t0.002193\t0.013997\t46.810\t-0.787\t-0.540\t63.434\t16.540\t0.189\t32.756\t6\n1050.00\t0.262\t0.000\t0.000309\t-126.260\t0.020\t72.702\t0.127\t-0.231\t0.002430\t0.015124\t39.355\t-0.832\t-0.610\t62.518\t19.461\t-0.127\t31.946\t6\n1040.00\t0.260\t0.000\t0.000318\t-125.964\t0.020\t75.031\t0.128\t0.385\t0.002484\t0.015566\t25.924\t-0.859\t-0.624\t63.496\t16.981\t0.216\t32.170\t6\n1030.00\t0.257\t0.188\t0.000307\t-126.777\t0.021\t73.109\t0.129\t-0.978\t0.002386\t0.014367\t-7.827\t-0.821\t-0.613\t65.162\t19.786\t-0.553\t32.348\t6\n1020.00\t0.255\t-0.223\t0.000332\t-125.645\t0.021\t74.086\t0.127\t0.780\t0.002609\t0.015732\t-9.855\t-0.898\t-0.644\t64.748\t18.466\t0.433\t31.910\t6\n1010.00\t0.252\t-0.205\t0.000326\t-122.426\t0.021\t74.850\t0.124\t0.582\t0.002625\t0.015691\t-12.979\t-0.917\t-0.583\t63.731\t17.260\t0.316\t31.125\t6\n1000.00\t0.250\t0.000\t0.000344\t-126.486\t0.021\t73.746\t0.125\t0.868\t0.002762\t0.016307\t-6.249\t-0.921\t-0.681\t64.664\t18.858\t0.473\t31.227\t6\n990.00\t0.248\t0.000\t0.000345\t-129.249\t0.021\t74.185\t0.121\t1.055\t0.002843\t0.016110\t-6.046\t-0.890\t-0.727\t65.452\t18.544\t0.561\t30.414\t6\n980.00\t0.245\t-0.006\t0.000303\t-127.584\t0.020\t70.345\t0.121\t-0.027\t0.002504\t0.014834\t7.825\t-0.801\t-0.617\t62.027\t22.162\t-0.015\t30.449\t6\n970.00\t0.243\t-0.237\t0.000352\t-127.903\t0.021\t72.136\t0.121\t1.071\t0.002907\t0.016707\t-4.551\t-0.926\t-0.721\t63.860\t20.583\t0.567\t30.394\t6\n960.00\t0.240\t0.020\t0.000301\t-134.758\t0.021\t75.245\t0.117\t0.412\t0.002578\t0.014046\t-23.209\t-0.711\t-0.705\t66.350\t17.479\t0.210\t29.262\t6\n950.00\t0.237\t0.000\t0.000306\t-129.798\t0.015\t71.993\t0.115\t-1.494\t0.002659\t0.019828\t-7.725\t-0.783\t-0.652\t46.999\t15.280\t-0.754\t28.849\t6\n940.00\t0.235\t0.151\t0.000307\t-117.301\t0.022\t73.328\t0.111\t1.049\t0.002758\t0.013727\t8.402\t-0.908\t-0.469\t68.593\t20.541\t0.510\t27.893\t6\n930.00\t0.233\t0.000\t0.000302\t-123.107\t0.020\t72.702\t0.110\t0.060\t0.002754\t0.014778\t12.313\t-0.844\t-0.550\t62.182\t19.356\t0.028\t27.533\t6\n920.00\t0.230\t-0.186\t0.000302\t-115.950\t0.020\t72.856\t0.113\t-0.764\t0.002671\t0.014975\t12.250\t-0.904\t-0.440\t61.254\t18.892\t-0.378\t28.318\t6\n910.00\t0.228\t0.162\t0.000380\t-118.295\t0.022\t74.509\t0.110\t0.736\t0.003444\t0.017511\t21.676\t-1.116\t-0.601\t66.543\t18.449\t0.356\t27.706\t6\n900.00\t0.225\t0.000\t0.000413\t-126.909\t0.020\t72.466\t0.104\t1.428\t0.003978\t0.020841\t34.670\t-1.101\t-0.827\t60.917\t19.241\t0.651\t26.051\t6\n890.00\t0.222\t0.112\t0.000307\t-138.724\t0.017\t72.345\t0.099\t-0.692\t0.003089\t0.018050\t22.012\t-0.674\t-0.768\t52.234\t16.625\t-0.300\t24.899\t6\n880.00\t0.220\t-0.205\t0.000363\t-118.059\t0.017\t89.319\t0.087\t15.897\t0.004152\t0.020958\t-1.844\t-1.067\t-0.569\t55.587\t0.660\t6.009\t21.087\t6\n870.00\t0.218\t-0.046\t0.000307\t-105.194\t0.022\t119.795\t0.106\t42.935\t0.002893\t0.013725\t-20.892\t-0.986\t-0.268\t61.990\t-35.500\t18.121\t19.477\t6\n860.00\t0.215\t-0.124\t0.000310\t-99.212\t0.030\t111.736\t0.144\t35.288\t0.002147\t0.010479\t-37.367\t-1.020\t-0.166\t87.808\t-35.022\t20.930\t29.567\t6\n850.00\t0.213\t0.087\t0.000389\t-117.554\t0.034\t98.591\t0.166\t25.675\t0.002346\t0.011562\t-53.526\t-1.151\t-0.600\t106.168\t-16.048\t18.044\t37.520\t6\n840.00\t0.210\t-0.145\t0.000442\t-108.534\t0.037\t92.653\t0.179\t18.896\t0.002470\t0.011803\t-77.454\t-1.397\t-0.469\t119.135\t-5.524\t14.544\t42.468\t6\n830.00\t0.207\t-0.166\t0.000441\t-113.571\t0.040\t80.925\t0.189\t6.603\t0.002332\t0.011022\t-78.391\t-1.346\t-0.587\t126.186\t20.167\t5.449\t47.079\t6\n820.00\t0.205\t0.143\t0.000540\t-118.455\t0.033\t60.359\t0.153\t-13.557\t0.003525\t0.016336\t-15.260\t-1.582\t-0.858\t91.963\t52.321\t-9.009\t37.361\t6\n810.00\t0.203\t0.200\t0.000405\t-127.908\t0.024\t58.618\t0.114\t-13.601\t0.003556\t0.016932\t75.220\t-1.065\t-0.829\t64.945\t39.625\t-6.716\t27.756\t6\n800.00\t0.200\t-0.008\t0.000398\t-124.827\t0.023\t60.562\t0.110\t-11.838\t0.003634\t0.017097\t92.039\t-1.089\t-0.758\t64.598\t36.443\t-5.639\t26.897\t6\n790.00\t0.198\t0.000\t0.000402\t-129.320\t0.022\t60.167\t0.100\t-11.700\t0.004012\t0.018500\t68.966\t-1.036\t-0.849\t60.026\t34.424\t-5.100\t24.620\t6\n780.00\t0.195\t0.000\t0.000386\t-132.523\t0.021\t62.474\t0.100\t-9.910\t0.003856\t0.018053\t55.481\t-0.949\t-0.871\t60.656\t31.623\t-4.323\t24.744\t6\n770.00\t0.192\t0.183\t0.000379\t-125.887\t0.021\t66.044\t0.099\t-7.553\t0.003820\t0.017694\t-2.619\t-1.022\t-0.740\t62.206\t27.637\t-3.268\t24.646\t6\n760.00\t0.190\t0.081\t0.000374\t-127.392\t0.020\t67.709\t0.091\t-4.828\t0.004095\t0.018579\t-25.538\t-0.991\t-0.757\t59.509\t24.404\t-1.932\t22.850\t6\n750.00\t0.187\t-0.095\t0.000301\t-125.041\t0.018\t68.214\t0.088\t-4.949\t0.003407\t0.016501\t-30.532\t-0.822\t-0.576\t54.240\t21.689\t-1.914\t22.096\t6\n740.00\t0.185\t-0.147\t0.000354\t-118.674\t0.020\t69.510\t0.092\t-5.526\t0.003852\t0.017597\t-15.848\t-1.036\t-0.567\t60.461\t22.588\t-2.225\t22.987\t6\n730.00\t0.183\t0.011\t0.000380\t-122.723\t0.020\t71.351\t0.091\t-2.675\t0.004159\t0.018593\t-1.334\t-1.066\t-0.685\t62.367\t21.057\t-1.071\t22.926\t6\n720.00\t0.180\t0.177\t0.000334\t-114.895\t0.019\t72.680\t0.086\t-3.510\t0.003877\t0.017674\t9.316\t-1.009\t-0.469\t58.182\t18.138\t-1.323\t21.566\t6\n710.00\t0.177\t0.171\t0.000388\t-110.308\t0.020\t74.059\t0.085\t-3.214\t0.004569\t0.019272\t10.862\t-1.213\t-0.449\t61.673\t17.620\t-1.194\t21.275\t6\n700.00\t0.175\t-0.068\t0.000522\t-117.944\t0.022\t71.746\t0.089\t-1.862\t0.005863\t0.023346\t24.044\t-1.536\t-0.815\t68.156\t22.488\t-0.726\t22.342\t6\n690.00\t0.172\t-0.069\t0.000401\t-127.057\t0.020\t69.208\t0.084\t-3.768\t0.004775\t0.020201\t6.039\t-1.065\t-0.804\t59.481\t22.580\t-1.382\t20.997\t6\n680.00\t0.170\t0.123\t0.000359\t-123.360\t0.019\t71.505\t0.083\t-2.791\t0.004346\t0.018694\t-0.597\t-0.999\t-0.658\t58.120\t19.449\t-1.008\t20.687\t6\n670.00\t0.168\t0.104\t0.000381\t-117.180\t0.020\t73.735\t0.082\t-2.043\t0.004620\t0.019195\t-6.959\t-1.129\t-0.579\t61.378\t17.913\t-0.737\t20.650\t6\n660.00\t0.165\t-0.137\t0.000375\t-116.038\t0.020\t74.784\t0.080\t0.115\t0.004657\t0.019209\t-19.718\t-1.122\t-0.548\t60.297\t16.405\t0.041\t20.198\t6\n650.00\t0.162\t-0.106\t0.000390\t-109.627\t0.020\t75.086\t0.079\t-2.714\t0.004926\t0.019973\t-25.722\t-1.223\t-0.437\t60.783\t16.191\t-0.940\t19.814\t6\n640.00\t0.160\t0.016\t0.000439\t-111.396\t0.020\t74.971\t0.078\t-0.385\t0.005657\t0.021445\t0.543\t-1.361\t-0.533\t63.737\t17.116\t-0.130\t19.453\t6\n630.00\t0.157\t0.157\t0.000519\t-112.802\t0.021\t74.383\t0.079\t1.324\t0.006565\t0.024264\t35.130\t-1.595\t-0.671\t65.655\t18.360\t0.459\t19.836\t6\n620.00\t0.155\t-0.009\t0.000523\t-119.361\t0.022\t72.356\t0.080\t-1.582\t0.006553\t0.024084\t26.971\t-1.520\t-0.855\t66.159\t21.038\t-0.553\t20.012\t6\n610.00\t0.153\t0.000\t0.000424\t-125.722\t0.020\t71.197\t0.076\t-3.521\t0.005576\t0.021055\t25.088\t-1.147\t-0.825\t61.095\t20.814\t-1.173\t19.061\t6\n600.00\t0.150\t0.000\t0.000445\t-120.861\t0.020\t73.691\t0.072\t-0.341\t0.006149\t0.022107\t-22.448\t-1.274\t-0.761\t61.551\t18.015\t-0.109\t18.190\t6\n590.00\t0.147\t0.126\t0.000464\t-108.116\t0.020\t78.041\t0.070\t3.713\t0.006636\t0.023037\t13.995\t-1.470\t-0.481\t63.376\t13.432\t1.135\t17.502\t6\n580.00\t0.145\t0.000\t0.000613\t-121.783\t0.022\t74.630\t0.076\t4.482\t0.008022\t0.028213\t31.242\t-1.736\t-1.075\t67.180\t18.474\t1.498\t19.108\t6\n570.00\t0.142\t0.000\t0.000324\t-108.463\t0.016\t82.304\t0.060\t12.294\t0.005388\t0.020209\t47.654\t-1.026\t-0.343\t50.596\t6.838\t3.215\t14.746\t6\n560.00\t0.140\t-0.127\t0.000628\t-122.014\t0.025\t63.408\t0.085\t-8.954\t0.007424\t0.025595\t-127.637\t-1.776\t-1.110\t70.229\t35.141\t-3.306\t20.971\t6\n550.00\t0.138\t0.000\t0.000599\t-103.464\t0.022\t74.438\t0.072\t-1.642\t0.008323\t0.026810\t-50.742\t-1.942\t-0.465\t68.605\t19.111\t-0.517\t18.047\t6\n540.00\t0.135\t0.135\t0.000679\t-110.435\t0.022\t72.828\t0.072\t-0.802\t0.009385\t0.030388\t-25.108\t-2.121\t-0.790\t68.596\t21.195\t-0.254\t18.138\t6\n530.00\t0.132\t-0.009\t0.000678\t-113.450\t0.024\t73.185\t0.073\t-2.087\t0.009245\t0.028705\t9.733\t-2.072\t-0.898\t72.717\t21.977\t-0.670\t18.379\t6\n520.00\t0.130\t-0.127\t0.000690\t-123.986\t0.021\t66.528\t0.066\t-5.933\t0.010404\t0.032705\t15.072\t-1.906\t-1.285\t62.300\t27.049\t-1.720\t16.545\t6\n510.00\t0.127\t0.000\t0.000633\t-133.643\t0.020\t63.490\t0.064\t-5.993\t0.009970\t0.032467\t17.507\t-1.528\t-1.458\t56.211\t28.030\t-1.666\t15.860\t6\n500.00\t0.125\t0.096\t0.000562\t-128.035\t0.019\t66.544\t0.064\t-5.982\t0.008767\t0.029288\t15.377\t-1.476\t-1.155\t56.788\t24.632\t-1.677\t16.000\t6\n@-Ecp%$\n\nDRV:        89 poly= xxxxx   Chip not enabled\n              galvo= 00000 00000 00000 00000 00000 00040 000ff 000ff 000ff 00099\n                  9= 00099 00099 0002f 00061 00000 0002a 0007f 00000\n\nDRV:        90 poly= xxxxx   Chip not enabled\n              galvo= 00000 00000 00000 00000 00070 00040 000ff 000ff 000ff 00099\n                  9= 00099 00099 0002f 00061 00000 0002a 0007f 00000\nLow=388376, High=393428, diff=5052, diffAllowed=38837\nAvg Motor I^2*R Loss=0.253906 W, Avg Current=0.356569 A\nAvg Following Error=3.7611 Deg\nPolarity Detect Attempts=0\nResistance=1.252 ohms\n        V1=0.124 volts, Cur1=0.124 amps\n        V2=0.251 volts, Cur2=0.226 amps\n       ETC=3275 uSec, Inductance=2485 uH\nMotor is UNKNOWN polarity, position is Inverted\nCurrent Offsets: Low= -55 (-0.01731 A)  High=30 (0.00944 A)\nMeasure positions: @start=     0, ~@tc1=-15474, @end1=-13955, ~@tc2=-13919, @end2=  6989\nHolding position inverted, current limit=1.00 ...  Hold failed, inrange = 0\nHolding position normal, current limit=1.00 ...  Polarity = normal, inrange=274\n\nS-->\nDRV:       206 poly= xxxxx   Chip not enabled\n              galvo= xxxxx   Chip not enabled\n\nS-->" ("input string")
  n1 = xnode "Match Regular Expression"("input string"="input Bode plot", "regular expression"="-CaP%[$]\\n") -> ("after match"=w25:string, "error out"=w2:errorcluster)  [unwired: 4 in, 3 out]
  n2 = xnode "Match Regular Expression"("input string"=w25, "regular expression"="\\n@-Ecp%[$]", "error in"=w2) -> ("before match"=w23:string, "error out"=→"error out":errorcluster)  [unwired: 3 in, 3 out]
  n3 = Spreadsheet String To Array(format string="%g", spreadsheet string=w23, array type (2D Dbl)=dbl[][] []) -> (array=w16:dbl[][])  [unwired: 1 in]
  n4 = Delete From Array(array=w16, index (row)=0) -> (array with subset deleted=w17:dbl[][])  [unwired: 2 in, 1 out]
  n5 = call "Sort 2D Array.vim"("index"=0, "dimension to index (column)"=enum16{"column", "row"}."column", "2D array"=w17) -> ("sorted 2D array"=w12:dbl[][])  [unwired: 7 in, 1 out]
  n6 = Index Array(array=w12, index (col) #1=0 ("disabled index (col)"), index (col) #2=9 ("index (col)"), index (col) #3=10 ("index (col)")) -> (element #1=w5:dbl[], element #2=w6:dbl[], element #3=w4:dbl[])  [unwired: 3 in]
  "FreqHz" <- w5
  "PosAmpVsPWM" <- w6
  "PosAmpVsCur" <- w4
  n7 = Build Array(w5, w6, w4) -> (w8:dbl[][])
  n8 = Bundle("sorted 2D array"=w5, "sorted 2D array"=w6) -> (w11:T2)  [unwired: 1 in]
  n9 = Bundle("sorted 2D array"=w5, "sorted 2D array"=w4) -> (w10:T2)  [unwired: 1 in]
  n10 = Transpose 2D Array(2D array=w8) -> (transposed array=→"Bode plot":dbl[][])
  n11 = Build Array(w11, w10) -> (→"XY Graph":T1)
